vi "QMH_Tester_rev1.vi"() -> ()   [LabVIEW 2015]
doc: "Demonstrates the fundamentals of the Queued Message Handler design pattern in LabVIEW. A queued message handler, in its simplest form, is composed of two loops. The Event Handling Loop responds to user interface events by enqueuing \"messages\" on a message queue. These messages are dequeued in the Message Handling Loop. Note that the Message Handling Loop is also capable of sending messages to itself."
uses:
  Controls/Control_Stop.ctl
  Controls/Control_Unitherm Connect Disconnect Bool.ctl
  Controls/Control_M4X Connect Disconnect Bool.ctl
  Controls/Control_Fornax Connect Disconnect Bool.ctl
  Controls/Control_Unitherm Set Load Numeric.ctl
  Controls/Control_Unitherm Set Load Bool.ctl
  Controls/Control_Unitherm VISA Resource.ctl
  Controls/Control_Unitherm Clear Load Bool.ctl
  Controls/Control_PXI-7854R Connect Disconnect Bool.ctl
  Controls/Control_PXI-7854R 75kHz Bool.ctl
  Controls/Control_PXI-7854R uSec Off Numeric.ctl
  Controls/Control_PXI-7854R uSec On Numeric.ctl
  Controls/Control_PXI-7854R Resource.ctl
  Controls/Control_PXI-7854R Set Config Bool.ctl
  Controls/Control_PXI-7854R Set Config Enum.ctl
  Controls/Control_M4X Read Current Bool.ctl
  Controls/Control_Log Bool.ctl
  Controls/Control_Fornax Ligasure Activate Port Bool.ctl
  Controls/Control_Fornax Bipolar Activate Port Bool.ctl
  Controls/Control_Fornax Bipolar Decrease Power.ctl
  Controls/Control_Fornax Bipolar Increase Power.ctl
  Controls/Control_Fornax Bipolar Enum.ctl
  Controls/Control_Fornax Mono1 Cut Activate Port Bool.ctl
  Controls/Control_Fornax Mono1 Cut Enum.ctl
  Controls/Control_Fornax Mono1 Cut Increase Power.ctl
  Controls/Control_Fornax Mono1 Cut Decrease Power.ctl
  Controls/Control_Fornax Mono1 Coag Enum.ctl
  Controls/Control_Fornax Mono1 Coag Activate Port Bool.ctl
  Controls/Control_Fornax Mono1 Coag Increase Power.ctl
  Controls/Control_Fornax Mono1 Coag Decrease Power.ctl
  Controls/Control_Fornax Mono2 Cut Activate Port Bool.ctl
  Controls/Control_Fornax Mono2 Cut Increase Power.ctl
  Controls/Control_Fornax Mono2 Cut Decrease Power.ctl
  Controls/Control_Fornax Mono2 Cut Enum.ctl
  Controls/Control_Fornax Mono2 Coag Activate Port Bool.ctl
  Controls/Control_Fornax Mono2 Coag Enum.ctl
  Controls/Control_Fornax Mono2 Coag Increase Power.ctl
  Controls/Control_Fornax Mono2 Coag Decrease Power.ctl
  Controls/QMH Fundamentals - Message Cluster.ctl
  Controls/Control_Message Handling Cluster.ctl
  Controls/Control_M4X Connection.ctl
  Controls/Control_PXI-7854R FPGA Reference.ctl
  Controls/Control_Config Cluster.ctl
  Controls/Control_Config Unitherm Port.ctl
  Controls/Control_Config Simulate Values.ctl
  Controls/Control_Log Queue.ctl
  Controls/Control_Log Cluster.ctl
  Controls/Control_Log Time.ctl
  Controls/Control_Log Waveform Cluster.ctl
  Controls/Control_Log Analysis Cluster.ctl
  Controls/Control_Log Flag.ctl
  Controls/Config_Stop Notifier Enum.ctl
  Controls/Control_Log Loop Cluster.ctl
  Controls/Control_Log TDMS Filename.ctl
  Controls/Control_Log t0.ctl
  Controls/Control_Unitherm Connect Disconnect Cluster.ctl
  Controls/Control_PXI-7854R Connect Disconnect Cluster.ctl
  Controls/Control_PXI-7854R Set Config Cluster.ctl
  Controls/Control_Fornax Generator.ctl
  Controls/Control_Fornax Energy Channel ID.ctl
  Controls/Control_Fornax Instrument Type.ctl
  Controls/Control_Fornax Parameter Type.ctl
  Controls/Control_Fornax Parameter Value.ctl
  Controls/Control_Fornax Energy Mode.ctl
  <vilib>/Utility/error.llb/Error Cluster From Error Code.vi
  <vilib>/rvi/errors/niLvFpgaAdjustHostInterfaceError.vi
  <vilib>/rvi/interface/nirviReadWriteControl/nirviReadWriteControl.xnode
  <vilib>/ErrorRing/Error Ring.xnode
  NiFpgaLv.dll
  <vilib>/rvi/interface/Simulation/niFpgaSimulationCallBeginRW.vi
panel:
  in  "Mono2 Coag minus":T1
  in  "Mono2 Coag plus":T2
  in  "Mono2 Coag Enum":T3=enum."Spray"
  in  "Mono2 Coag Activate":T4
  in  "Mono2 Cut Enum":T5
  in  "Mono2 Cut minus":T6
  in  "Mono2 Cut plus":T7
  in  "Mono2 Cut Activate":T8
  in  "Mono1 Coag minus":T9
  in  "Mono1 Coag plus":T10
  in  "Mono1 Coag Activate":T11
  in  "Mono1 Coag Enum":T12=enum."Spray"
  in  "Mono1 Cut minus":T13
  in  "Mono1 Cut plus":T14
  in  "Mono1 Cut Enum":T15
  in  "Mono1 Cut Activate":T16
  in  "Bipolar Enum":T17
  in  "Bipolar plus":T18
  in  "Bipolar minus":T19
  in  "Bipolar Activate":T20
  in  "Ligasure Activate":T21
  out "Logging?":bool
  in  "Log?":T22
  out "Data":waveform(dbl)[](graph)
  out "Array":T23(array[cluster])
  in  "Read Current":T24
  in  "7854 Config Enum":T25=enum."Off"
  in  "7854 Set Config":T26
  in  "resource name":T27="PXI1Slot6" caption="RIO Device"
  in  "uSec On":T28=7
  in  "uSec Off":T29=6
  in  "75kHz":T30=TRUE
  in  "7854 Connect/Disconnect":T31
  out "PXI-7854R Connected?":bool
  in  "Clear Load":T32
  in  "Unitherm Refnum in":T33="COM4"
  in  "Set Load":T34
  in  "Load (Ohms)":T35
  out "M4X Connected?":bool
  in  "Fornax Connect/Disconnect":T36
  in  "M4X Connect/Disconnect":T37
  in  "Unitherm Connect/Disconnect":T38
  out "Unitherm Connected?":bool
  out "Fornax Connected?":bool
  out "Display Message":string="\"Stop\" button pressed"
  in  "Stop":T39
  # "Unitherm"
  # "PXI-7854R"
  # "M4X"
  # "Note: If you are creating a LabVIEW application based on the Queued Message Handler design pattern, create a Queued Message Handler project from the File > Create Project dialog."
  # "Fornax"
  # "Mono1"
  # "Mono2"
  # "Bipolar"
  # "Ligasure"
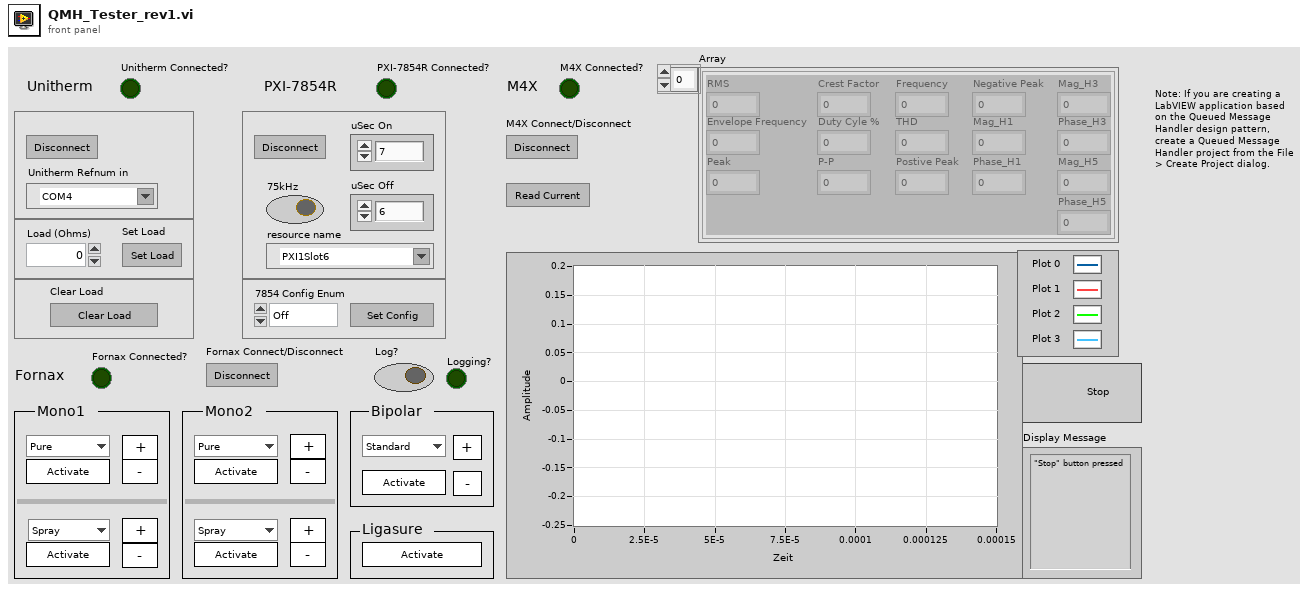
[diagram p1: front panel]
types:
  T1 = typedef "Control_Fornax Mono2 Coag Decrease Power.ctl" = bool
  T2 = typedef "Control_Fornax Mono2 Coag Increase Power.ctl" = bool
  T3 = typedef "Control_Fornax Mono2 Coag Enum.ctl" = enum16{"Fulgerate", "Spray"}
  T4 = typedef "Control_Fornax Mono2 Coag Activate Port Bool.ctl" = bool
  T5 = typedef "Control_Fornax Mono2 Cut Enum.ctl" = enum16{"Pure", "Blend"}
  T6 = typedef "Control_Fornax Mono2 Cut Decrease Power.ctl" = bool
  T7 = typedef "Control_Fornax Mono2 Cut Increase Power.ctl" = bool
  T8 = typedef "Control_Fornax Mono2 Cut Activate Port Bool.ctl" = bool
  T9 = typedef "Control_Fornax Mono1 Coag Decrease Power.ctl" = bool
  T10 = typedef "Control_Fornax Mono1 Coag Increase Power.ctl" = bool
  T11 = typedef "Control_Fornax Mono1 Coag Activate Port Bool.ctl" = bool
  T12 = typedef "Control_Fornax Mono1 Coag Enum.ctl" = enum16{"Fulgerate", "Spray"}
  T13 = typedef "Control_Fornax Mono1 Cut Decrease Power.ctl" = bool
  T14 = typedef "Control_Fornax Mono1 Cut Increase Power.ctl" = bool
  T15 = typedef "Control_Fornax Mono1 Cut Enum.ctl" = enum16{"Pure", "Blend"}
  T16 = typedef "Control_Fornax Mono1 Cut Activate Port Bool.ctl" = bool
  T17 = typedef "Control_Fornax Bipolar Enum.ctl" = enum16{"Standard", "Macro", "Precision"}
  T18 = typedef "Control_Fornax Bipolar Increase Power.ctl" = bool
  T19 = typedef "Control_Fornax Bipolar Decrease Power.ctl" = bool
  T20 = typedef "Control_Fornax Bipolar Activate Port Bool.ctl" = bool
  T21 = typedef "Control_Fornax Ligasure Activate Port Bool.ctl" = bool
  T22 = typedef "Control_Log Bool.ctl" = bool
  T23 = cluster{"RMS":dbl, "Envelope Frequency":dbl, "Peak":dbl, "Crest Factor":dbl, "Duty Cyle %":dbl, "P-P":dbl, "Frequency":dbl, "THD":dbl, "Postive Peak":dbl, "Negative Peak":dbl, "Mag_H1":dbl, "Phase_H1":dbl, "Mag_H3":dbl, "Phase_H3":dbl, "Mag_H5":dbl, "Phase_H5":dbl}[]
  T24 = typedef "Control_M4X Read Current Bool.ctl" = bool
  T25 = typedef "Control_PXI-7854R Set Config Enum.ctl" = enum16{"Mono 1", "Mono 2", "BiPolar", "LigaSure", "Off"}
  T26 = typedef "Control_PXI-7854R Set Config Bool.ctl" = bool
  T27 = typedef "Control_PXI-7854R Resource.ctl" = tag
  T28 = typedef "Control_PXI-7854R uSec On Numeric.ctl" = u16
  T29 = typedef "Control_PXI-7854R uSec Off Numeric.ctl" = u16
  T30 = typedef "Control_PXI-7854R 75kHz Bool.ctl" = bool
  T31 = typedef "Control_PXI-7854R Connect Disconnect Bool.ctl" = bool
  T32 = typedef "Control_Unitherm Clear Load Bool.ctl" = bool
  T33 = typedef "Control_Unitherm VISA Resource.ctl" = refnum<visa-resource-name>
  T34 = typedef "Control_Unitherm Set Load Bool.ctl" = bool
  T35 = typedef "Control_Unitherm Set Load Numeric.ctl" = i32
  T36 = typedef "Control_Fornax Connect Disconnect Bool.ctl" = bool
  T37 = typedef "Control_M4X Connect Disconnect Bool.ctl" = bool
  T38 = typedef "Control_Unitherm Connect Disconnect Bool.ctl" = bool
  T39 = typedef "Control_Stop.ctl" = bool
  T40 = typedef "Control_Log Loop Cluster.ctl" = cluster{"tdms file out":T41, "t0":T42}
  T41 = typedef "Control_Log TDMS Filename.ctl" = refnum<k34>
  T42 = typedef "Control_Log t0.ctl" = string
  T43 = typedef "Config_Stop Notifier Enum.ctl" = enum16{"Initialize", "Read Notifier", "Notify", "Close"}
  T44 = typedef "Control_Log Cluster.ctl" = cluster{"Log Time":T45, "Log Waveform Cluster":T46, "Log Analysis Cluster":T47}
  T45 = typedef "Control_Log Time.ctl" = timestamp
  T46 = typedef "Control_Log Waveform Cluster.ctl" = waveform(dbl)
  T47 = typedef "Control_Log Analysis Cluster.ctl" = cluster{"RMS":dbl, "Envelope Frequency":dbl, "Peak":dbl, "Crest Factor":dbl, "Duty Cyle %":dbl, "P-P":dbl, "Frequency":dbl, "THD":dbl, "Postive Peak":dbl, "Negative Peak":dbl, "Mag_H1":dbl, "Phase_H1":dbl, "Mag_H3":dbl, "Phase_H3":dbl, "Mag_H5":dbl, "Phase_H5":dbl}
  T48 = typedef "Control_Message Handling Cluster.ctl" = cluster{"Fornax Connected?":refnum<vi>, "Unitherm Connected?":refnum<vi>, "M4X Connected?":refnum<vi>, "Unitherm Connect/Disconnect":refnum<vi>, "Fornax Connection":refnum<k5>, "UNITHERM Connection":refnum<visa-resource-name>, "M4X Connection":T49, "PXI-7854R FPGA Reference":T50, "PXI-7854R Connected?":refnum<vi>, "Fornax Connect/Disconnect":refnum<vi>, "7854 Connect/Disconnect":refnum<vi>, "M4X Connect/Disconnect":refnum<vi>, "Config Cluster":T51, "Log Queue":T54, "Log Analysis Cluster":T47, "Log Waveform Cluster":T46, "Log Time":T45, "Log Flag":T55}
  T49 = typedef "Control_M4X Connection.ctl" = u32
  T50 = typedef "Control_PXI-7854R FPGA Reference.ctl" = refnum<k20>
  T51 = typedef "Control_Config Cluster.ctl" = cluster{"Unitherm Port":T52, "Simulate Values":T53}
  T52 = typedef "Control_Config Unitherm Port.ctl" = string
  T53 = typedef "Control_Config Simulate Values.ctl" = bool
  T54 = typedef "Control_Log Queue.ctl" = refnum<queue>
  T55 = typedef "Control_Log Flag.ctl" = bool
  T56 = typedef "QMH Fundamentals - Message Cluster.ctl" = cluster{"Message":string, "Message Data":variant}
  T57 = typedef "Control_Unitherm Connect Disconnect Cluster.ctl" = cluster{"Unitherm Connect/Disconnect":T38, "Unitherm Refnum in":T33}
  T58 = typedef "Control_PXI-7854R Connect Disconnect Cluster.ctl" = cluster{"PXI-7854R Resource":T27, "75kHz":T30, "uSec Off":T29, "uSec On":T28, "7854 Connect/Disconnect":T31}
  T59 = typedef "Control_PXI-7854R Set Config Cluster.ctl" = cluster{"7854 Config Enum":T25, "7854 Set Config":T26}
  T60 = typedef "Control_Fornax Energy Mode.ctl" = enum16{"SPRAY_MODE", "CUT_MODE", "BLEND_MODE", "FULGERATE_MODE", "BIPOLAR_MODE", "VESSEL_SEALING_MODE", "VALLEYLAB_MODE", "BIPOLAR_RESECTION_CUT_MODE", "BIPOLAR_RESECTION_COAG_MODE", "AUTOBIPOLAR_MODE", "VIPER_HLA", "SOFT_COAG_MODE", "ECUT_MODE", "SHARED_SPRAY_MODE", "SHARED_FULGERATE_MODE", "CARDIO_MONO_MODE", "CARDIO_BIPOLAR_MODE", "BIPOLAR_LOW_MODE", "BIPOLAR_MACRO_MODE", "BIPOLAR_STANDARD_MODE", "BIPOLAR_MEDIUM_MODE", "VL_ENDOSCOPY_MODE", "NUM_ENERGY_MODES"}
  T61 = typedef "Control_Fornax Parameter Value.ctl" = i32
  T62 = typedef "Control_Fornax Parameter Type.ctl" = enum16{"POWER_PARAMETER", "CUT_MODALITY_POWER_PARAMETER", "COAG_MODALITY_POWER_PARAMETER", "VL_MODALITY_POWER_PARAMETER", "BY_MODE_POWER_PARAMETER", "VL_ENDO_CUT_MODALITY_POWER_PARAMETER", "VL_ENDO_COAG_MODALITY_POWER_PARAMETER", "VL_ENDO_COAG_ON_CUT_MODALITY_POWER_PARAMETER", "MODE_PARAMETER   (for changing Bipolar mode)", "CUT_MODALITY_MODE_PARAMETER  (for changing monopolar cut mode)", "COAG_MODALITY_MODE_PARAMETER (for changing monopolar coag mode)", "VL_ENDO_COAG_MODALITY_MODE_PARAMETER", "VL_ENDO_CUT_INTERVAL_PARAMETER", "VL_ENDO_CUT_DURATION_PARAMETER", "POWER_BAR_PARAMETER", "MAX_ACTIVATION_MSEC_TIME_PARAMETER", "AUTOBIPOLAR_DELAY_MSEC_TIME", "VL_ENDO_COAG_QUICK_ACCESS_PARAMETER"}
  T63 = typedef "Control_Fornax Instrument Type.ctl" = enum16{"INSTRUMENT_TYPE_UNKNOWN", "INSTRUMENT_TYPE_MONOPOLAR", "INSTRUMENT_TYPE_BIPOLAR", "INSTRUMENT_TYPE_TRIVERSE", "INSTRUMENT_TYPE_LIGASURE", "INSTRUMENT_TYPE_ADVANCE_II", "INSTRUMENT_TYPE_BIPOLAR_RESECTION", "INSTRUMENT_TYPE_HOOK", "INSTRUMENT_TYPE_BIZACT", "INSTRUMENT_TYPE_CARDIOBLATE_BIP", "INSTRUMENT_TYPE_CARDIOBLATE_BIP_GEMINI_S", "INSTRUMENT_TYPE_CARDIOBLATE_MONO", "INSTRUMENT_TYPE_ULTRASONIC", "INSTRUMENT_TYPE_MONOPOLAR_GI ", "INSTRUMENT_TYPE_GOLDILOCKS "}
  T64 = typedef "Control_Fornax Energy Channel ID.ctl" = enum16{"EC_MONO_1  ", "EC_BIPOLAR  ", "EC_MONO_2  ", "EC_ADVANCED  ", "EC_ADVANCED_ECUT  ", "EC_ADVANCED_DCUT  ", "EC_SHARED_COAG  ", "EC_INTERNAL_BIP_CAL  "}
  T65 = typedef "Control_Fornax Generator.ctl" = string
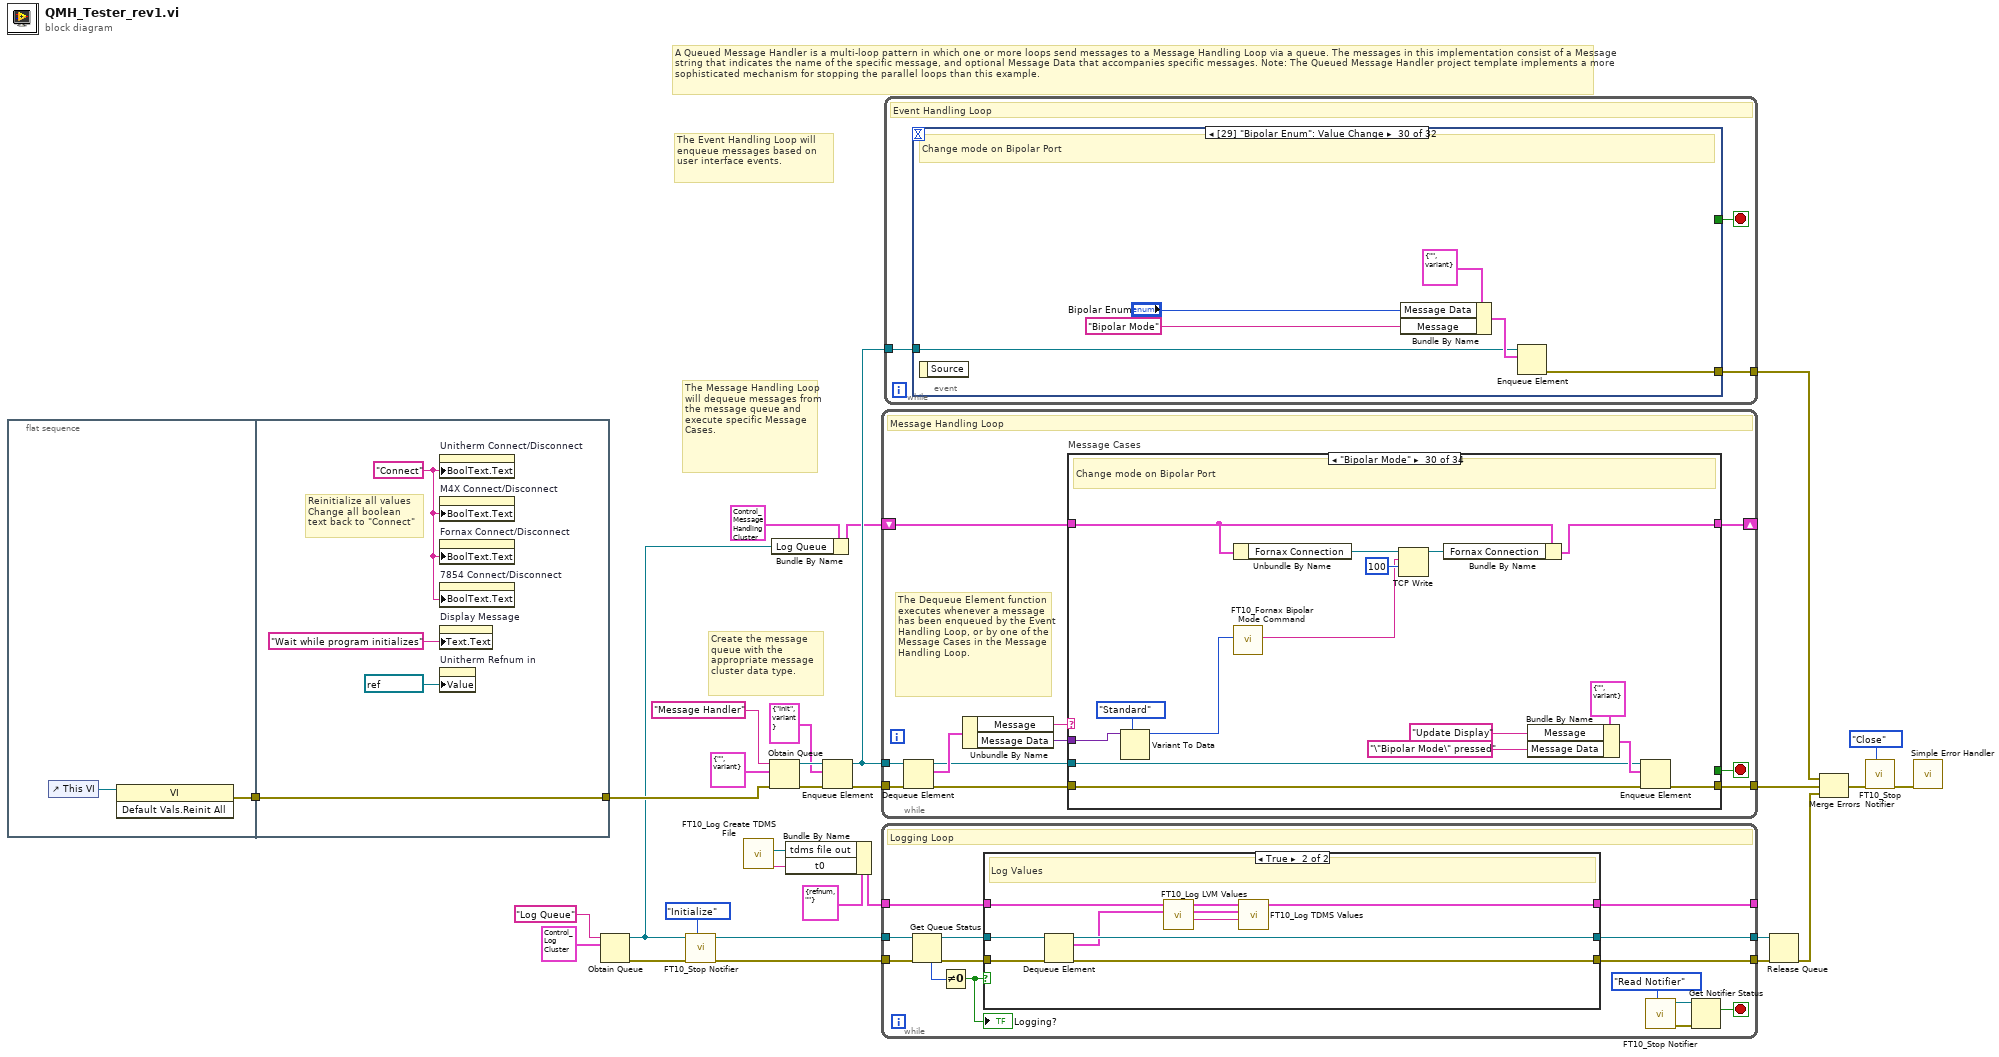
[diagram p0: block diagram]
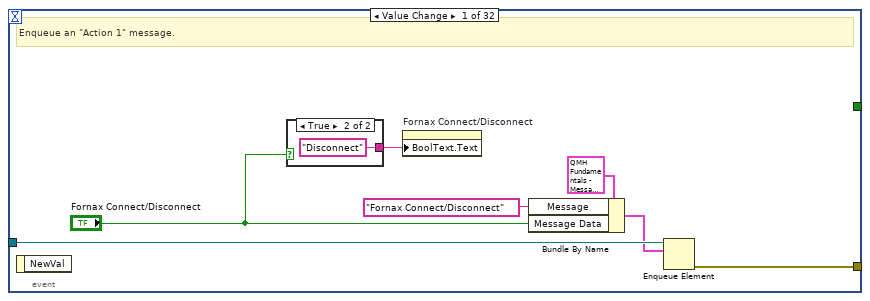
[diagram p3: hidden frame]
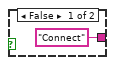
[diagram p4: hidden frame]
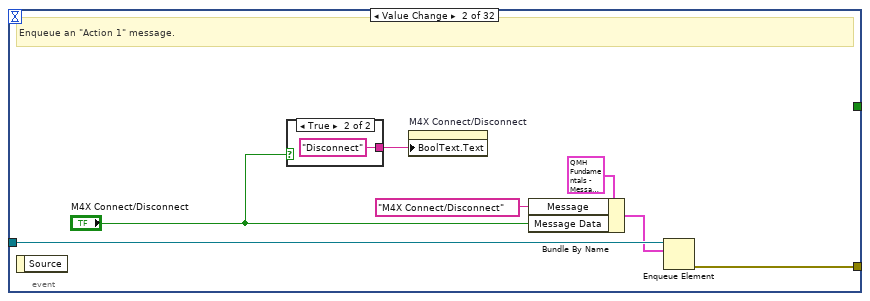
[diagram p5: hidden frame]
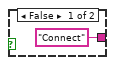
[diagram p6: hidden frame]
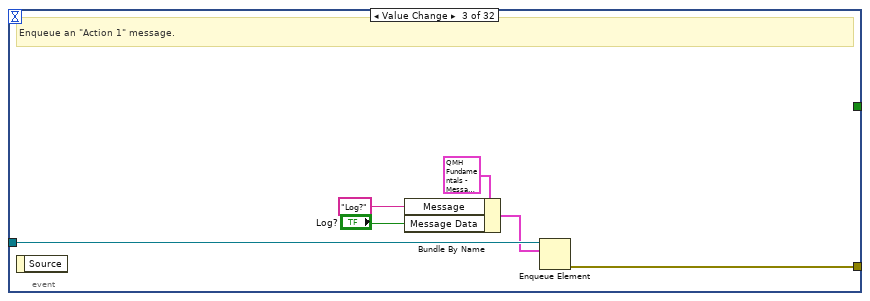
[diagram p7: hidden frame]
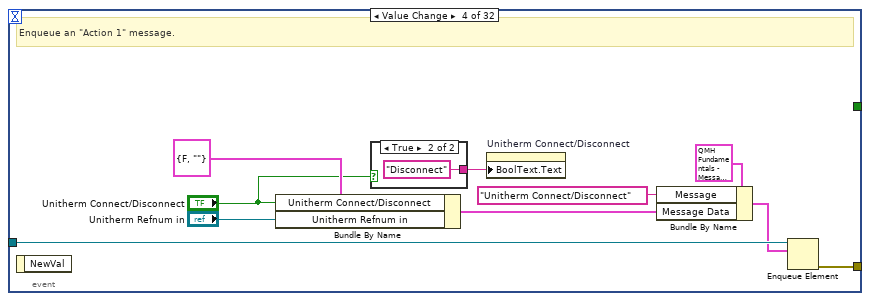
[diagram p8: hidden frame]
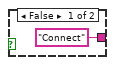
[diagram p9: hidden frame]
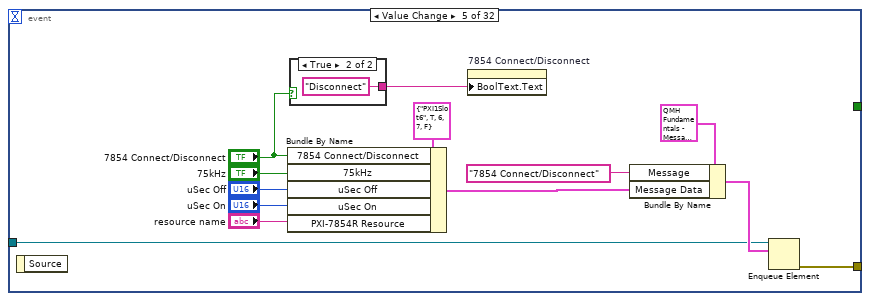
[diagram p10: hidden frame]
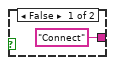
[diagram p11: hidden frame]
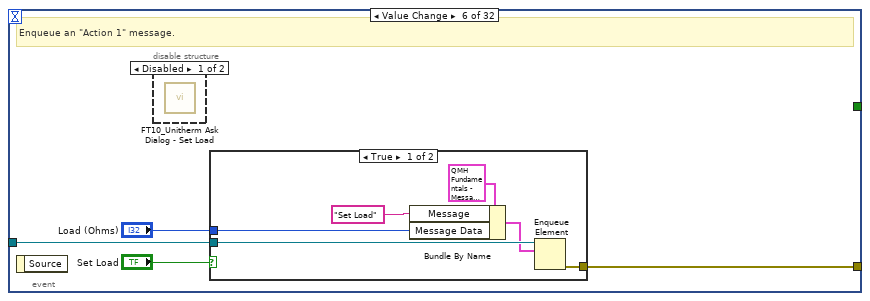
[diagram p12: hidden frame]
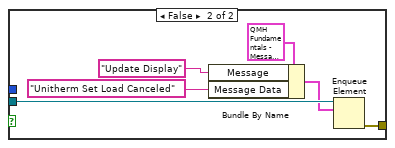
[diagram p14: hidden frame]
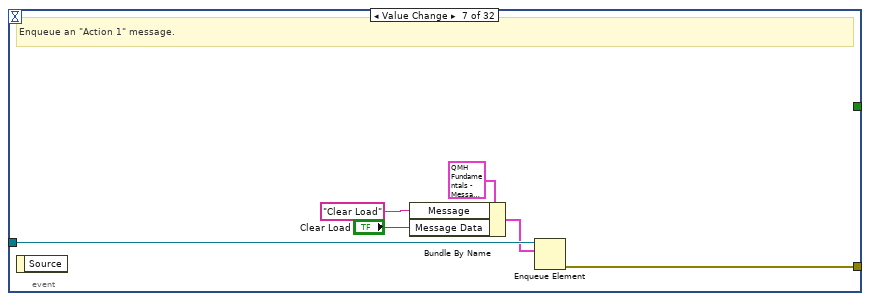
[diagram p15: hidden frame]
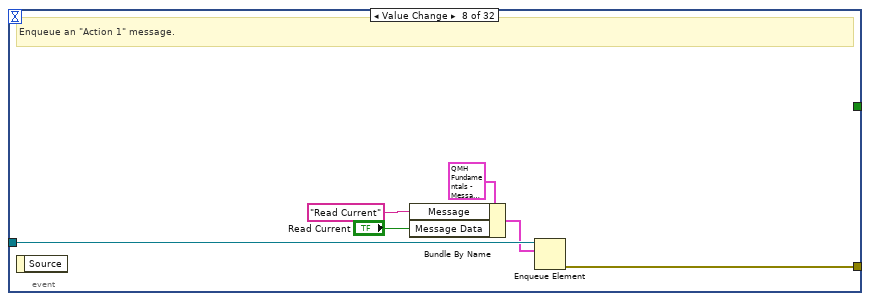
[diagram p16: hidden frame]
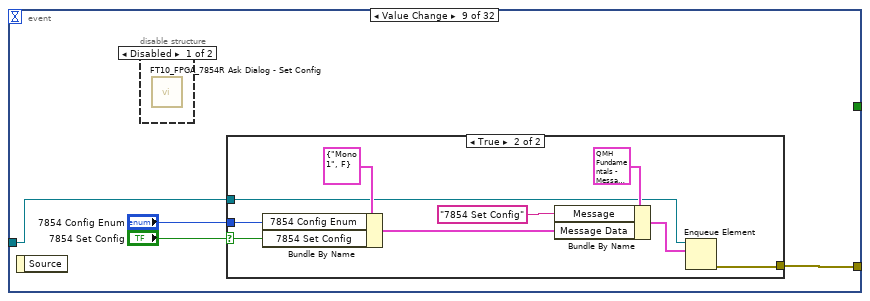
[diagram p17: hidden frame]
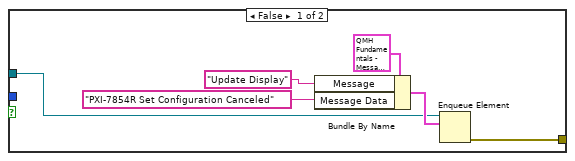
[diagram p19: hidden frame]
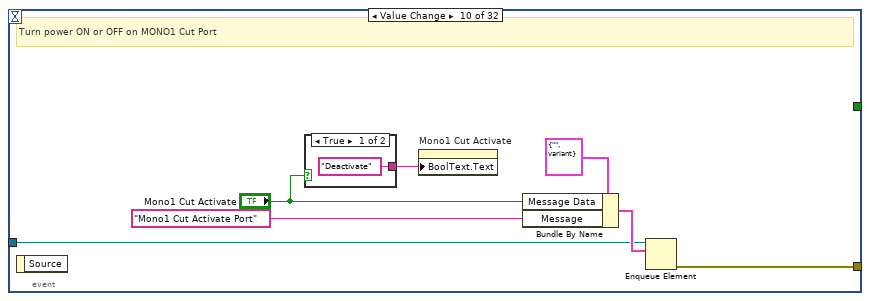
[diagram p20: hidden frame]
diagram:
  # "Create the message queue with the appropriate message cluster data type."
  # "A Queued Message Handler is a multi-loop pattern in which one or more loops send messages to a Message Handling Loop via a queue. The messages in this implementation consist of a Message string that indicates the name of the specific message, and optional Message Data that accompanies specific messages. Note: The Queued Message Handler project template implements a more sophisticated mechanism for stopping the parallel loops than this example."
  # "The Message Handling Loop will dequeue messages from the message queue and execute specific Message Cases."
  # "The Event Handling Loop will enqueue messages based on user interface events."
  n1 = flat-sequence {
    tunnel: [w30] -> w18
    tunnel: [w35] -> w21
    tunnel: w18 -> [w35]
    frame #0 {
      n2 = control-ref of="This VI"() -> (w31:refnum<vi>)
      n3 = invoke class="VI" method="Default Vals.Reinit All"(reference=w31) -> (error out=w30:errorcluster)  [unwired: 2 in, 2 out]
    }
    frame #1 {
      w33 = "Connect" ("Boolean Text.Text")
      # "Reinitialize all values\nChange all boolean\ntext back to \"Connect\""
      n4 = property on="Unitherm Connect/Disconnect" class="Bool (strict)"("BoolText.Text"=w33) -> ()  [unwired: 2 in, 2 out]
      n5 = property on="M4X Connect/Disconnect" class="Bool (strict)"("BoolText.Text"=w33) -> ()  [unwired: 2 in, 2 out]
      n6 = property on="Fornax Connect/Disconnect" class="Bool (strict)"("BoolText.Text"=w33) -> ()  [unwired: 2 in, 2 out]
      n7 = property on="7854 Connect/Disconnect" class="Bool (strict)"("BoolText.Text"=w33) -> ()  [unwired: 2 in, 2 out]
      n8 = property on="Display Message" class="Str"("Text.Text"="Wait while program initializes" ("Display Message")) -> ()  [unwired: 2 in, 2 out]
      n9 = property on="Unitherm Refnum in" class="VISAName (strict)"("Value"=refnum<visa-resource-name> "COM4" ("Unitherm Refnum in")) -> ()  [unwired: 2 in, 2 out]
    }
  }
  n10 = Obtain Queue(name (unnamed)="Log Queue", element data type=T44 {"Log Time"=timestamp(0 s since 1904-01-01), "Log Waveform Cluster"={"t0"=timestamp(0 s since 1904-01-01), "dt"=1.0, "Y"=[]}, "Log Analysis Cluster"={"RMS"=0.0, "Envelope Frequency"=0.0, "Peak"=0.0, "Crest Factor"=0.0, "Duty Cyle %"=0.0, "P-P"=0.0, "Frequency"=0.0, "THD"=0.0, "Postive Peak"=0.0, "Negative Peak"=0.0, "Mag_H1"=0.0, "Phase_H1"=0.0, "Mag_H3"=0.0, "Phase_H3"=0.0, "Mag_H5"=0.0, "Phase_H5"=0.0}}) -> (queue out=w11:refnum<queue>, error out=w9:errorcluster)  [unwired: 3 in, 1 out]
  n11 = call "FT10_Stop Notifier.vi"("Selector"=Config_Stop_Notifier_Enum."Initialize", "error in (no error)"=w9) -> ("error out"=w8:errorcluster)  [unwired: 8 in, 1 out]
  n12 = call "FT10_Log Create TDMS File.vi"() -> ("t0"=w2:T42, "tdms file out"=w1:T41)  [unwired: 10 in]
  n13 = Obtain Queue(name (unnamed)="Message Handler", element data type=T56 {"Message"="", "Message Data"=variant} ("Message Cluster"), error in (no error)=w21) -> (queue out=w25:refnum<queue>, error out=w26:errorcluster)  [unwired: 2 in, 1 out]
  n14 = Bundle By Name(cluster=T48 {"Fornax Connected?"=refnum, "Unitherm Connected?"=refnum, "M4X Connected?"=refnum, "Unitherm Connect/Disconnect"=refnum, "Fornax Connection"=refnum, "UNITHERM Connection"="", "M4X Connection"=0, "PXI-7854R FPGA Reference"=refnum, "PXI-7854R Connected?"=refnum, "Fornax Connect/Disconnect"=refnum, "7854 Connect/Disconnect"=refnum, "M4X Connect/Disconnect"=refnum, "Config Cluster"={"Unitherm Port"="COM4", "Simulate Values"=TRUE}, "Log Queue"=refnum, "Log Analysis Cluster"={"RMS"=0.0, "Envelope Frequency"=0.0, "Peak"=0.0, "Crest Factor"=0.0, "Duty Cyle %"=0.0, "P-P"=0.0, "Frequency"=0.0, "THD"=0.0, "Postive Peak"=0.0, "Negative Peak"=0.0, "Mag_H1"=0.0, "Phase_H1"=0.0, "Mag_H3"=0.0, "Phase_H3"=0.0, "Mag_H5"=0.0, "Phase_H5"=0.0}, "Log Waveform Cluster"={"t0"=timestamp(0 s since 1904-01-01), "dt"=1.0, "Y"=[]}, "Log Time"=timestamp(0 s since 1904-01-01), "Log Flag"=FALSE}, "Log Queue"=w11) -> (w12:T48)
  n15 = Bundle By Name(cluster=T40 {"tdms file out"=refnum, "t0"=""}, "tdms file out"=w1, "t0"=w2) -> (w3:T40)
  n16 = Enqueue Element(queue=w25, element=T56 {"Message"="Init", "Message Data"=variant}, error in (no error)=w26) -> (queue out=w19:refnum<queue>, error out=w24:errorcluster)  [unwired: 1 in, 1 out]
  n17 = while {
    tunnel: w19 -> [w45]
    tunnel: w24 -> [w46]
    tunnel: [w38] -> w29
    shift-right: [w39] -> _
    shift-left: w12 -> [w36]
    stop <- w37 stop-if-true
    # "The Dequeue Element function executes whenever a message has been enqueued by the Event Handling Loop, or by one of the Message Cases in the Message Handling Loop."
    # "Message Handling Loop"
    n18 = Dequeue Element(queue=w45, error in (no error)=w46) -> (queue out=w43:refnum<queue>, element=w44:T56, error out=w42:errorcluster)  [unwired: 1 in, 1 out]
    n19 = Unbundle By Name(w44) -> ("Message"=w41:string, "Message Data"=w40:variant)
    n20 = case "Message Cases" shown="\"Bipolar Mode\"" w41 {
      selector: w41 -> [_ _ _ _ _ _ _ _ _ _ _ _ _ _ _ _ _ _ _ _ _ _ _ _ _ _ _ _ _ _ _ _ _ w610]
      tunnel: w43 -> [w68 w85 w104 w133 w152 w177 w190 w203 w204 w232 w246 w260 w274 w288 w302 w321 w340 w359 w378 w397 w416 w435 w454 w473 w492 w508 w524 w540 w556 w572 _ _ w604 _]
      tunnel: w42 -> [w47 w84 w95 w124 w143 w163 w179 w195 w207 w231 w245 w259 w273 w287 w301 w320 w339 w358 w377 w396 w415 w434 w453 w472 w491 w507 w523 w539 w555 w571 w582 w588 w596 w609]
      tunnel: [w69 w86 w105 w134 w153 w169 w183 w197 w208 w230 w244 w258 w272 w286 w300 w319 w338 w357 w376 w395 w414 w433 w452 w471 w490 w506 w522 w538 w554 w570 w582 w585 w589 w609] -> w38
      tunnel: w40 -> [_ w79 w102 w123 w144 w167 _ _ w216 w227 w242 w256 w268 w282 w296 _ _ _ _ _ _ _ _ _ _ w499 w515 w530 w547 w563 w581 w587 _ _]
      tunnel: w36 -> [w67 w90 w97 w128 w146 w170 w184 w198 w219 w229 w243 w257 w271 w285 w299 w318 w337 w356 w375 w394 w413 w432 w451 w470 w489 w505 w521 w537 w553 w569 w580 w583 w599 w607]
      tunnel: [w62 w83 w96 w127 w145 w171 w185 w191 w218 w223 w241 w255 w270 w284 w298 w317 w336 w355 w374 w393 w412 w431 w450 w469 w488 w504 w520 w536 w552 w568 w579 w583 w598 w607] -> w39
      tunnel: [_ _ _ _ _ _ _ _ _ _ _ _ _ _ _ _ _ _ _ _ _ _ _ _ _ _ _ _ _ _ _ _ TRUE _] -> w37
      frame "Init" {
        # "Initialize - Create reference for connection indicators. Connect to Fornax, M4X, and Unitherm."
        n21 = call "FT10_Config Parse File.vi"("error in (no error)"=w47, "File Path Control"=path "Config.ini") -> ("error out"=w49:errorcluster, "Config cluster"=w48:T51)  [unwired: 8 in]
        n22 = control-ref of="Fornax Connected?"() -> (w66:refnum<vi>)
        n23 = control-ref of="Unitherm Connected?"() -> (w65:refnum<vi>)
        n24 = control-ref of="M4X Connected?"() -> (w64:refnum<vi>)
        n25 = control-ref of="PXI-7854R Connected?"() -> (w56:refnum<vi>)
        n26 = control-ref of="Unitherm Connect/Disconnect"() -> (w54:refnum<vi>)
        n27 = control-ref of="Fornax Connect/Disconnect"() -> (w53:refnum<vi>)
        n28 = control-ref of="7854 Connect/Disconnect"() -> (w52:refnum<vi>)
        n29 = control-ref of="M4X Connect/Disconnect"() -> (w51:refnum<vi>)
        n30 = Bundle By Name(cluster=w67, "Fornax Connected?"=w66, "Unitherm Connected?"=w65, "M4X Connected?"=w64, "PXI-7854R Connected?"=w56, "UNITHERM Connection"=refnum<visa-resource-name> "COM4", "Unitherm Connect/Disconnect"=w54, "Fornax Connect/Disconnect"=w53, "7854 Connect/Disconnect"=w52, "M4X Connect/Disconnect"=w51, "Config Cluster"=w48) -> (w63:T48)
        n31 = Bundle By Name(cluster=T56 {"Message"="", "Message Data"=variant} ("Message Cluster"), "Message"="Update Display", "Message Data"="Initialize Complete" ("L10n_Action 1 Pressed")) -> (w72:T56)
        n32 = call "FT10_Connect Hardware.vi"("Message Handling Cluster in"=w63, "error in (no error)"=w49) -> ("Message Handling Cluster out"=w62:T48, "Fornax Connected?"=→"Fornax Connected?":bool, "Unitherm Connected?"=→"Unitherm Connected?":bool, "M4X Connected?"=→"M4X Connected?":bool, "PXI-7854R Connected?"=→"PXI-7854R Connected?":bool, "error out"=w61:errorcluster)  [unwired: 8 in]
        n33 = Enqueue Element(queue=w68, element=w72, error in (no error)=w47) -> (error out=w70:errorcluster)  [unwired: 1 in, 2 out]
        n34 = Merge Errors(w61, w70) -> (w69:errorcluster)
      }
      frame "Fornax Connect/Disconnect" {
        # "Connect or disconnect from Fornax."
        n35 = Variant To Data(type=TRUE, Variant=w79) -> (data=w76:bool)  [unwired: 1 in, 1 out]
        n36 = case shown="True" w76 {
          tunnel: ["Fornax Disconnect" ("L10n_Action 1 Pressed") "Fornax Connect" ("L10n_Action 1 Pressed")] -> w75
          frame False {
          }
          frame True {
          }
        }
        n37 = call "FT10_Connect Fornax Handler.vi"("error in (no error)"=w84, "Message Data"=w79, "Message Handling Cluster in"=w90) -> ("error out"=w81:errorcluster, "Fornax Connected?"=w80:bool, "Message Handling Cluster out"=w83:T48)  [unwired: 6 in]
        n38 = Bundle By Name(cluster=T56 {"Message"="", "Message Data"=variant} ("Message Cluster"), "Message Data"=w75, "Message"="Update Display") -> (w88:T56)
        n39 = Enqueue Element(queue=w85, element=w88, error in (no error)=w84) -> (error out=w87:errorcluster)  [unwired: 1 in, 2 out]
        n40 = Unbundle By Name(w83) -> ("Fornax Connected?"=w82:refnum<vi>)
        n41 = property class="Bool (strict)"(reference=w82, "Value"=w80) -> ()  [unwired: 1 in, 2 out]
        n42 = Merge Errors(w81, w87) -> (w86:errorcluster)
      }
      frame "M4X Connect/Disconnect" {
        # "Connect or disconnect from M4X."
        n43 = Variant To Data(type=TRUE, Variant=w102) -> (data=w99:bool)  [unwired: 1 in, 1 out]
        n44 = case shown="True" w99 {
          tunnel: ["M4X Disconnect" ("L10n_Action 1 Pressed") "M4X Connect" ("L10n_Action 1 Pressed")] -> w98
          tunnel: w97 -> [w111 w117]
          tunnel: [w111 w116] -> w96
          tunnel: w95 -> [w110 w115]
          tunnel: [w110 w114] -> w94
          tunnel: [FALSE ("M4X Connected?") w113] -> w93
          frame False {
          }
          frame True {
            n45 = call "FT10_Connect M4X.vi"("error in (no error)"=w115, "reset device"=TRUE, "Board #"=u32 0, "Message Handling Cluster in"=w117) -> ("error out"=w114:errorcluster, "M4X Connected?"=w113:bool, "Message Handling Cluster out"=w116:T48)  [unwired: 4 in, 1 out]
          }
        }
        n46 = Bundle By Name(cluster=T56 {"Message"="", "Message Data"=variant} ("Message Cluster"), "Message Data"=w98, "Message"="Update Display") -> (w107:T56)
        n47 = Enqueue Element(queue=w104, element=w107, error in (no error)=w95) -> (error out=w106:errorcluster)  [unwired: 1 in, 2 out]
        n48 = Unbundle By Name(w96) -> ("M4X Connected?"=w103:refnum<vi>)
        n49 = property class="Bool (strict)"(reference=w103, "Value"=w93) -> ()  [unwired: 1 in, 2 out]
        n50 = Merge Errors(w94, w106) -> (w105:errorcluster)
      }
      frame "Unitherm Connect/Disconnect" {
        # "Connect or disconnect from Unitherm."
        n51 = Variant To Data(type=T57 {"Unitherm Connect/Disconnect"=FALSE, "Unitherm Refnum in"=""}, Variant=w123) -> (data=w130:T57)  [unwired: 1 in, 1 out]
        n52 = Unbundle By Name(w130) -> ("Unitherm Connect/Disconnect"=w121:T38)
        n53 = call "FT10_Connect Unitherm Handler.vi"("error in (no error)"=w124, "Message Data"=w123, "Message Handling Cluster in"=w128) -> ("error out"=w125:errorcluster, "Unitherm Connected?"=w126:bool, "Message Handling Cluster out"=w127:T48)  [unwired: 6 in]
        n54 = case shown="False" w121 {
          tunnel: ["Unitherm Disconnect" ("L10n_Action 1 Pressed") "Unitherm Connect" ("L10n_Action 1 Pressed")] -> w129
          frame False {
          }
          frame True {
          }
        }
        n55 = Unbundle By Name(w127) -> ("Unitherm Connected?"=w132:refnum<vi>)
        n56 = Bundle By Name(cluster=T56 {"Message"="", "Message Data"=variant} ("Message Cluster"), "Message Data"=w129, "Message"="Update Display") -> (w136:T56)
        n57 = Enqueue Element(queue=w133, element=w136, error in (no error)=w124) -> (error out=w135:errorcluster)  [unwired: 1 in, 2 out]
        n58 = property class="Bool (strict)"(reference=w132, "Value"=w126) -> ()  [unwired: 1 in, 2 out]
        n59 = Merge Errors(w125, w135) -> (w134:errorcluster)
      }
      frame "7854 Connect/Disconnect" {
        # "Connect or disconnect from Unitherm."
        n60 = Variant To Data(type=T58 {"PXI-7854R Resource"="PXI1Slot6", "75kHz"=TRUE, "uSec Off"=6, "uSec On"=7, "7854 Connect/Disconnect"=FALSE}, Variant=w144) -> (data=w149:T58)  [unwired: 1 in, 1 out]
        n61 = Unbundle By Name(w149) -> ("7854 Connect/Disconnect"=w147:T31)
        n62 = case shown="False" w147 {
          tunnel: ["PXI-7854R Disconnected" ("L10n_Action 1 Pressed") "PXI-7854R Connected" ("L10n_Action 1 Pressed")] -> w148
          frame False {
          }
          frame True {
          }
        }
        n63 = call "FT10_Connect FPGA_7854R Handler.vi"("error in"=w143, "Message Data"=w144, "Message Handling Cluster in"=w146) -> ("error out"=w142:errorcluster, "PXI-7854R Connected?"=w141:bool, "Message Handling Cluster out"=w145:T48)  [unwired: 6 in]
        n64 = Unbundle By Name(w145) -> ("PXI-7854R Connected?"=w151:refnum<vi>)
        n65 = Bundle By Name(cluster=T56 {"Message"="", "Message Data"=variant} ("Message Cluster"), "Message Data"=w148, "Message"="Update Display") -> (w155:T56)
        n66 = Enqueue Element(queue=w152, element=w155, error in (no error)=w143) -> (error out=w154:errorcluster)  [unwired: 1 in, 2 out]
        n67 = property class="Bool (strict)"(reference=w151, "Value"=w141) -> ()  [unwired: 1 in, 2 out]
        n68 = Merge Errors(w142, w154) -> (w153:errorcluster)
      }
      frame "Set Load" {
        # "Adjust the Impedance of the Unitherm."
        n69 = Variant To Data(type=0 ("Load (Ohms)"), Variant=w167) -> (data=w162:i32)  [unwired: 1 in, 1 out]
        n70 = Number To Decimal String(number=w162) -> (decimal integer string=w160:string)  [unwired: 1 in]
        n71 = Unbundle By Name(w170) -> ("UNITHERM Connection"=w166:refnum<visa-resource-name>)
        n72 = Concatenate Strings("Unitherm Load set to " ("L10n_Action 1 Pressed"), w160, " Ohms" ("string")) -> (w161:string)
        n73 = call "FT10_Unitherm Set Load.vi"("error in (no error)"=w163, "Load Impedance"=w162, "VISA Refnum in"=w166) -> ("error out"=w164:errorcluster, "VISA Refnum out"=w165:refnum<visa-resource-name>)  [unwired: 7 in]
        n74 = Bundle By Name(cluster=T56 {"Message"="", "Message Data"=variant} ("Message Cluster"), "Message"="Update Display", "Message Data"=w161) -> (w173:T56)
        n75 = Bundle By Name(cluster=w170, "UNITHERM Connection"=w165) -> (w171:T48)
        n76 = Enqueue Element(queue=w177, element=w173, error in (no error)=w163) -> (error out=w176:errorcluster)  [unwired: 1 in, 2 out]
        n77 = Merge Errors(w164, w176) -> (w169:errorcluster)
      }
      frame "Clear Load" {
        # "Adjust the Impedance of the Unitherm."
        n78 = Unbundle By Name(w184) -> ("UNITHERM Connection"=w181:refnum<visa-resource-name>)
        n79 = call "FT10_Unitherm Clear Load.vi"("error in (no error)"=w179, "VISA Refnum in"=w181) -> ("error out"=w178:errorcluster, "VISA Refnum out"=w180:refnum<visa-resource-name>)  [unwired: 8 in]
        n80 = Bundle By Name(cluster=T56 {"Message"="", "Message Data"=variant} ("Message Cluster"), "Message"="Update Display", "Message Data"="Unitherm Load Cleared" ("L10n_Action 1 Pressed")) -> (w186:T56)
        n81 = Bundle By Name(cluster=w184, "UNITHERM Connection"=w180) -> (w185:T48)
        n82 = Enqueue Element(queue=w190, element=w186, error in (no error)=w179) -> (error out=w189:errorcluster)  [unwired: 1 in, 2 out]
        n83 = Merge Errors(w178, w189) -> (w183:errorcluster)
      }
      frame "Read Current" {
        # "Read data from M4X and send to logging loop if logging is enabled."
        n84 = call "FT10_M4X Read.vi"("Message Handling Cluster in"=w198) -> ("Waveform Array"=→"Data":waveform(dbl)[], "Analysis Cluster Array"=→"Array":T23, "Message Handling Cluster out"=w192:T48)  [unwired: 8 in]
        n85 = Bundle By Name(cluster=T56 {"Message"="", "Message Data"=variant} ("Message Cluster"), "Message"="Update Display", "Message Data"="\"Read Current\" pressed" ("L10n_Action 1 Pressed")) -> (w199:T56)
        n86 = call "FT10_Log Queue Data.vi"("Message Handling Cluster in"=w192) -> ("Message Handling Cluster out"=w191:T48)  [unwired: 10 in]
        n87 = Enqueue Element(queue=w203, element=w199, error in (no error)=w195) -> (error out=w202:errorcluster)  [unwired: 1 in, 2 out]
        n88 = Merge Errors(w202) -> (w197:errorcluster)
      }
      frame "7854 Set Config" {
        n89 = Variant To Data(type=T59 {"7854 Config Enum"=enum."Mono 1", "7854 Set Config"=FALSE}, Variant=w216) -> (data=w221:T59)  [unwired: 1 in, 1 out]
        n90 = Unbundle By Name(w221) -> ("7854 Config Enum"=w215:T25)
        n91 = Unbundle By Name(w219) -> ("PXI-7854R FPGA Reference"=w220:T50)
        n92 = call "FT10_FPGA_7854R Set Config.vi"("7854 Config Enum"=w215) -> ("Config string"=w206:string, "Conn2/DIO_8_15 In"=w213:bool[], "Conn2/DIO_0_7 In"=w214:bool[])  [unwired: 8 in]
        n93 = xnode "Read/Write Control"("FPGA VI Reference In"=w220, "Conn2/DIO_0_7 In"=w214, "Conn2/DIO_8_15 In"=w213) -> ("FPGA VI Reference Out"=w217:T50)  [unwired: 1 in, 1 out]
        n94 = Concatenate Strings("PXI-7854R Configuration Set to " ("Display Message"), w206) -> (w205:string)
        n95 = Bundle By Name(cluster=w219, "PXI-7854R FPGA Reference"=w217) -> (w218:T48)
        n96 = Bundle By Name(cluster=T56 {"Message"="", "Message Data"=variant} ("Message Cluster"), "Message"="Update Display", "Message Data"=w205) -> (w209:T56)
        n97 = Enqueue Element(queue=w204, element=w209, error in (no error)=w207) -> (error out=w208:errorcluster)  [unwired: 1 in, 2 out]
      }
      frame "Mono1 Cut Activate Port" {
        # "Turn power ON or OFF on MONO1 Cut Port"
        n98 = Variant To Data(type=T16 FALSE ("Mono1 Cut Activate"), Variant=w227) -> (data=w224:T16)  [unwired: 1 in, 1 out]
        n99 = Unbundle By Name(w229) -> ("Fornax Connection"=w226:refnum<k5>)
        n100 = call "FT10_Fornax Mono1 Cut Activate Port Command.vi"("Mono1 Cut Activate"=w224, "TCP Network Connection in"=w226) -> ("TCP Network Connection out"=w225:refnum<k5>)  [unwired: 9 in]
        n101 = Bundle By Name(cluster=w229, "Fornax Connection"=w225) -> (w223:T48)
        n102 = Bundle By Name(cluster=T56 {"Message"="", "Message Data"=variant} ("Message Cluster"), "Message"="Update Display", "Message Data"="\"Mono1 Cut Activate Port\" pressed" ("L10n_Action 1 Pressed")) -> (w234:T56)
        n103 = Enqueue Element(queue=w232, element=w234, error in (no error)=w231) -> (error out=w230:errorcluster)  [unwired: 1 in, 2 out]
      }
      frame "Mono2 Cut Activate Port" {
        # "Turn power ON or OFF on MONO2 Cut Port"
        n104 = Variant To Data(type=T8 FALSE ("Mono2 Cut Activate"), Variant=w242) -> (data=w237:T8)  [unwired: 1 in, 1 out]
        n105 = Unbundle By Name(w243) -> ("Fornax Connection"=w239:refnum<k5>)
        n106 = call "FT10_Fornax Mono2 Cut Activate Port Command.vi"("Mono2 Cut Activate"=w237, "TCP Network Connection in"=w239) -> ("TCP Network Connection out"=w238:refnum<k5>)  [unwired: 9 in]
        n107 = Bundle By Name(cluster=w243, "Fornax Connection"=w238) -> (w241:T48)
        n108 = Bundle By Name(cluster=T56 {"Message"="", "Message Data"=variant} ("Message Cluster"), "Message"="Update Display", "Message Data"="\"Mono2 Cut Activate Port\" pressed" ("L10n_Action 1 Pressed")) -> (w248:T56)
        n109 = Enqueue Element(queue=w246, element=w248, error in (no error)=w245) -> (error out=w244:errorcluster)  [unwired: 1 in, 2 out]
      }
      frame "Mono1 Coag Activate Port" {
        # "Turn power ON or OFF on MONO1 Coag Port"
        n110 = Variant To Data(type=T11 FALSE ("Mono1 Coag Activate"), Variant=w256) -> (data=w251:T11)  [unwired: 1 in, 1 out]
        n111 = Unbundle By Name(w257) -> ("Fornax Connection"=w253:refnum<k5>)
        n112 = call "FT10_Fornax Mono1 Coag Activate Port Command.vi"("Mono1 Coag Activate"=w251, "TCP Network Connection in"=w253) -> ("TCP Network Connection out"=w252:refnum<k5>)  [unwired: 9 in]
        n113 = Bundle By Name(cluster=w257, "Fornax Connection"=w252) -> (w255:T48)
        n114 = Bundle By Name(cluster=T56 {"Message"="", "Message Data"=variant} ("Message Cluster"), "Message"="Update Display", "Message Data"="\"Mono1 Coag Activate Port\" pressed" ("L10n_Action 1 Pressed")) -> (w262:T56)
        n115 = Enqueue Element(queue=w260, element=w262, error in (no error)=w259) -> (error out=w258:errorcluster)  [unwired: 1 in, 2 out]
      }
      frame "Mono2 Coag Activate Port" {
        # "Turn power ON or OFF on MONO2 Coag Port"
        n116 = Variant To Data(type=T4 FALSE ("Mono2 Coag Activate"), Variant=w268) -> (data=w265:T4)  [unwired: 1 in, 1 out]
        n117 = Unbundle By Name(w271) -> ("Fornax Connection"=w267:refnum<k5>)
        n118 = call "FT10_Fornax Mono2 Coag Activate Port Command.vi"("Mono2 Coag Activate"=w265, "TCP Network Connection in"=w267) -> ("TCP Network Connection out"=w266:refnum<k5>)  [unwired: 9 in]
        n119 = Bundle By Name(cluster=w271, "Fornax Connection"=w266) -> (w270:T48)
        n120 = Bundle By Name(cluster=T56 {"Message"="", "Message Data"=variant} ("Message Cluster"), "Message"="Update Display", "Message Data"="\"Mono2 Coag Activate Port\" pressed" ("L10n_Action 1 Pressed")) -> (w276:T56)
        n121 = Enqueue Element(queue=w274, element=w276, error in (no error)=w273) -> (error out=w272:errorcluster)  [unwired: 1 in, 2 out]
      }
      frame "Ligasure Activate Port" {
        # "Turn power ON or OFF on Ligasure Port"
        n122 = Variant To Data(type=T21 FALSE ("Ligasure Activate"), Variant=w282) -> (data=w279:T21)  [unwired: 1 in, 1 out]
        n123 = Unbundle By Name(w285) -> ("Fornax Connection"=w281:refnum<k5>)
        n124 = call "FT10_Fornax Ligasure Activate Port Command.vi"("Ligasure Activate"=w279, "TCP Network Connection in"=w281) -> ("TCP Network Connection out"=w280:refnum<k5>)  [unwired: 9 in]
        n125 = Bundle By Name(cluster=w285, "Fornax Connection"=w280) -> (w284:T48)
        n126 = Bundle By Name(cluster=T56 {"Message"="", "Message Data"=variant} ("Message Cluster"), "Message"="Update Display", "Message Data"="\"Ligasure Activate Port\" pressed" ("L10n_Action 1 Pressed")) -> (w290:T56)
        n127 = Enqueue Element(queue=w288, element=w290, error in (no error)=w287) -> (error out=w286:errorcluster)  [unwired: 1 in, 2 out]
      }
      frame "Bipolar Activate Port" {
        # "Turn power ON or OFF on Bipolar Port"
        n128 = Variant To Data(type=T20 FALSE ("Bipolar Activate"), Variant=w296) -> (data=w293:T20)  [unwired: 1 in, 1 out]
        n129 = Unbundle By Name(w299) -> ("Fornax Connection"=w295:refnum<k5>)
        n130 = call "FT10_Fornax Bipolar Activate Port Command.vi"("Bipolar Activate"=w293, "TCP Network Connection in"=w295) -> ("TCP Network Connection out"=w294:refnum<k5>)  [unwired: 9 in]
        n131 = Bundle By Name(cluster=w299, "Fornax Connection"=w294) -> (w298:T48)
        n132 = Bundle By Name(cluster=T56 {"Message"="", "Message Data"=variant} ("Message Cluster"), "Message"="Update Display", "Message Data"="\"Bipolar Activate Port\" pressed" ("L10n_Action 1 Pressed")) -> (w304:T56)
        n133 = Enqueue Element(queue=w302, element=w304, error in (no error)=w301) -> (error out=w300:errorcluster)  [unwired: 1 in, 2 out]
      }
      frame "Mono1 Cut Decrease Power" {
        # "Decrease Mono1 Cut Power"
        # "Turn power level down on MONO1 Cut Port"
        n134 = Unbundle By Name(w318) -> ("Fornax Connection"=w309:refnum<k5>)
        n135 = call "FT10_Fornax Energy Parameter Command.vi"("Energy Channel ID"=Control_Fornax_Energy_Channel_ID."EC_MONO_1  ", "Generator"=T65 "CAMM_EXT_1234321_AJ1428000", "Instrument Type"=Control_Fornax_Instrument_Type."INSTRUMENT_TYPE_MONOPOLAR", "Parameter Type"=Control_Fornax_Parameter_Type."CUT_MODALITY_POWER_PARAMETER", "Parameter Value"=T61 2, "Energy Mode"=Control_Fornax_Energy_Mode."CUT_MODE") -> ("JSON Command"=w307:string)  [unwired: 9 in]
        n136 = TCP Write(connection ID=w309, data in=w307, 9:100 ("timeout ms (25000)")) -> (connection ID out=w308:refnum<k5>)  [unwired: 1 in, 2 out]
        n137 = Bundle By Name(cluster=w318, "Fornax Connection"=w308) -> (w317:T48)
        n138 = Bundle By Name(cluster=T56 {"Message"="", "Message Data"=variant} ("Message Cluster"), "Message"="Update Display", "Message Data"="\"Mono1 Cut Decrease Power\" pressed" ("L10n_Action 1 Pressed")) -> (w323:T56)
        n139 = Enqueue Element(queue=w321, element=w323, error in (no error)=w320) -> (error out=w319:errorcluster)  [unwired: 1 in, 2 out]
      }
      frame "Mono2 Cut Decrease Power" {
        # "Decrease Mono2 Cut Power"
        # "Turn power level down on MONO2 Cut Port"
        n140 = Unbundle By Name(w337) -> ("Fornax Connection"=w334:refnum<k5>)
        n141 = call "FT10_Fornax Energy Parameter Command.vi"("Energy Channel ID"=Control_Fornax_Energy_Channel_ID."EC_MONO_2  ", "Generator"=T65 "CAMM_EXT_1234321_AJ1428000", "Instrument Type"=Control_Fornax_Instrument_Type."INSTRUMENT_TYPE_MONOPOLAR", "Parameter Type"=Control_Fornax_Parameter_Type."CUT_MODALITY_POWER_PARAMETER", "Parameter Value"=T61 2, "Energy Mode"=Control_Fornax_Energy_Mode."CUT_MODE") -> ("JSON Command"=w326:string)  [unwired: 9 in]
        n142 = TCP Write(connection ID=w334, data in=w326, 9:100 ("timeout ms (25000)")) -> (connection ID out=w333:refnum<k5>)  [unwired: 1 in, 2 out]
        n143 = Bundle By Name(cluster=w337, "Fornax Connection"=w333) -> (w336:T48)
        n144 = Bundle By Name(cluster=T56 {"Message"="", "Message Data"=variant} ("Message Cluster"), "Message"="Update Display", "Message Data"="\"Mono2 Cut Decrease Power\" pressed" ("L10n_Action 1 Pressed")) -> (w342:T56)
        n145 = Enqueue Element(queue=w340, element=w342, error in (no error)=w339) -> (error out=w338:errorcluster)  [unwired: 1 in, 2 out]
      }
      frame "Mono1 Coag Decrease Power" {
        # "Decrease Mono1 Coag Power"
        # "Turn power level down on MONO1 Coag Port"
        n146 = Unbundle By Name(w356) -> ("Fornax Connection"=w353:refnum<k5>)
        n147 = call "FT10_Fornax Energy Parameter Command.vi"("Energy Channel ID"=Control_Fornax_Energy_Channel_ID."EC_MONO_1  ", "Generator"=T65 "CAMM_EXT_1234321_AJ1428000", "Instrument Type"=Control_Fornax_Instrument_Type."INSTRUMENT_TYPE_MONOPOLAR", "Parameter Type"=Control_Fornax_Parameter_Type."COAG_MODALITY_POWER_PARAMETER", "Parameter Value"=T61 2, "Energy Mode"=Control_Fornax_Energy_Mode."FULGERATE_MODE") -> ("JSON Command"=w345:string)  [unwired: 9 in]
        n148 = TCP Write(connection ID=w353, data in=w345, 9:100 ("timeout ms (25000)")) -> (connection ID out=w352:refnum<k5>)  [unwired: 1 in, 2 out]
        n149 = Bundle By Name(cluster=w356, "Fornax Connection"=w352) -> (w355:T48)
        n150 = Bundle By Name(cluster=T56 {"Message"="", "Message Data"=variant} ("Message Cluster"), "Message"="Update Display", "Message Data"="\"Mono1 Coag Decrease Power\" pressed" ("L10n_Action 1 Pressed")) -> (w361:T56)
        n151 = Enqueue Element(queue=w359, element=w361, error in (no error)=w358) -> (error out=w357:errorcluster)  [unwired: 1 in, 2 out]
      }
      frame "Mono2 Coag Decrease Power" {
        # "Decrease Mono2 Coag Power"
        # "Turn power level down on MONO2 Coag Port"
        n152 = Unbundle By Name(w375) -> ("Fornax Connection"=w372:refnum<k5>)
        n153 = call "FT10_Fornax Energy Parameter Command.vi"("Energy Channel ID"=Control_Fornax_Energy_Channel_ID."EC_MONO_2  ", "Generator"=T65 "CAMM_EXT_1234321_AJ1428000", "Instrument Type"=Control_Fornax_Instrument_Type."INSTRUMENT_TYPE_MONOPOLAR", "Parameter Type"=Control_Fornax_Parameter_Type."COAG_MODALITY_POWER_PARAMETER", "Parameter Value"=T61 2, "Energy Mode"=Control_Fornax_Energy_Mode."FULGERATE_MODE") -> ("JSON Command"=w364:string)  [unwired: 9 in]
        n154 = TCP Write(connection ID=w372, data in=w364, 9:100 ("timeout ms (25000)")) -> (connection ID out=w371:refnum<k5>)  [unwired: 1 in, 2 out]
        n155 = Bundle By Name(cluster=w375, "Fornax Connection"=w371) -> (w374:T48)
        n156 = Bundle By Name(cluster=T56 {"Message"="", "Message Data"=variant} ("Message Cluster"), "Message"="Update Display", "Message Data"="\"Mono2 Coag Decrease Power\" pressed" ("L10n_Action 1 Pressed")) -> (w380:T56)
        n157 = Enqueue Element(queue=w378, element=w380, error in (no error)=w377) -> (error out=w376:errorcluster)  [unwired: 1 in, 2 out]
      }
      frame "Bipolar Decrease Power" {
        # "Decrease Bipolar Power"
        # "Turn power level down on Bipolar Port"
        n158 = Unbundle By Name(w394) -> ("Fornax Connection"=w391:refnum<k5>)
        n159 = call "FT10_Fornax Energy Parameter Command.vi"("Energy Channel ID"=Control_Fornax_Energy_Channel_ID."EC_BIPOLAR  ", "Generator"=T65 "CAMM_EXT_1234321_AJ1428000", "Instrument Type"=Control_Fornax_Instrument_Type."INSTRUMENT_TYPE_BIPOLAR", "Parameter Type"=Control_Fornax_Parameter_Type."POWER_PARAMETER", "Parameter Value"=T61 2, "Energy Mode"=Control_Fornax_Energy_Mode."BIPOLAR_MODE") -> ("JSON Command"=w383:string)  [unwired: 9 in]
        n160 = TCP Write(connection ID=w391, data in=w383, 9:100 ("timeout ms (25000)")) -> (connection ID out=w390:refnum<k5>)  [unwired: 1 in, 2 out]
        n161 = Bundle By Name(cluster=w394, "Fornax Connection"=w390) -> (w393:T48)
        n162 = Bundle By Name(cluster=T56 {"Message"="", "Message Data"=variant} ("Message Cluster"), "Message"="Update Display", "Message Data"="\"Bipolar Decrease Power\" pressed" ("L10n_Action 1 Pressed")) -> (w399:T56)
        n163 = Enqueue Element(queue=w397, element=w399, error in (no error)=w396) -> (error out=w395:errorcluster)  [unwired: 1 in, 2 out]
      }
      frame "Mono1 Cut Increase Power" {
        # "Increase Mono1 Cut Power"
        # "Turn power level up on MONO1 Cut Port"
        n164 = Unbundle By Name(w413) -> ("Fornax Connection"=w410:refnum<k5>)
        n165 = call "FT10_Fornax Energy Parameter Command.vi"("Energy Channel ID"=Control_Fornax_Energy_Channel_ID."EC_MONO_1  ", "Generator"=T65 "CAMM_EXT_1234321_AJ1428000", "Instrument Type"=Control_Fornax_Instrument_Type."INSTRUMENT_TYPE_MONOPOLAR", "Parameter Type"=Control_Fornax_Parameter_Type."CUT_MODALITY_POWER_PARAMETER", "Parameter Value"=T61 1, "Energy Mode"=Control_Fornax_Energy_Mode."CUT_MODE") -> ("JSON Command"=w402:string)  [unwired: 9 in]
        n166 = TCP Write(connection ID=w410, data in=w402, 9:100 ("timeout ms (25000)")) -> (connection ID out=w409:refnum<k5>)  [unwired: 1 in, 2 out]
        n167 = Bundle By Name(cluster=w413, "Fornax Connection"=w409) -> (w412:T48)
        n168 = Bundle By Name(cluster=T56 {"Message"="", "Message Data"=variant} ("Message Cluster"), "Message"="Update Display", "Message Data"="\"Mono1 Cut Increase Power\" pressed" ("L10n_Action 1 Pressed")) -> (w418:T56)
        n169 = Enqueue Element(queue=w416, element=w418, error in (no error)=w415) -> (error out=w414:errorcluster)  [unwired: 1 in, 2 out]
      }
      frame "Mono2 Cut Increase Power" {
        # "Increase Mono2 Cut Power"
        # "Turn power level up on MONO2 Cut Port"
        n170 = Unbundle By Name(w432) -> ("Fornax Connection"=w429:refnum<k5>)
        n171 = call "FT10_Fornax Energy Parameter Command.vi"("Energy Channel ID"=Control_Fornax_Energy_Channel_ID."EC_MONO_2  ", "Generator"=T65 "CAMM_EXT_1234321_AJ1428000", "Instrument Type"=Control_Fornax_Instrument_Type."INSTRUMENT_TYPE_MONOPOLAR", "Parameter Type"=Control_Fornax_Parameter_Type."CUT_MODALITY_POWER_PARAMETER", "Parameter Value"=T61 1, "Energy Mode"=Control_Fornax_Energy_Mode."CUT_MODE") -> ("JSON Command"=w421:string)  [unwired: 9 in]
        n172 = TCP Write(connection ID=w429, data in=w421, 9:100 ("timeout ms (25000)")) -> (connection ID out=w428:refnum<k5>)  [unwired: 1 in, 2 out]
        n173 = Bundle By Name(cluster=w432, "Fornax Connection"=w428) -> (w431:T48)
        n174 = Bundle By Name(cluster=T56 {"Message"="", "Message Data"=variant} ("Message Cluster"), "Message"="Update Display", "Message Data"="\"Mono2 Cut Increase Power\" pressed" ("L10n_Action 1 Pressed")) -> (w437:T56)
        n175 = Enqueue Element(queue=w435, element=w437, error in (no error)=w434) -> (error out=w433:errorcluster)  [unwired: 1 in, 2 out]
      }
      frame "Mono1 Coag Increase Power" {
        # "Increase Mono1 Coag Power"
        # "Turn power level up on MONO1 Coag Port"
        n176 = Unbundle By Name(w451) -> ("Fornax Connection"=w448:refnum<k5>)
        n177 = call "FT10_Fornax Energy Parameter Command.vi"("Energy Channel ID"=Control_Fornax_Energy_Channel_ID."EC_MONO_1  ", "Generator"=T65 "CAMM_EXT_1234321_AJ1428000", "Instrument Type"=Control_Fornax_Instrument_Type."INSTRUMENT_TYPE_MONOPOLAR", "Parameter Type"=Control_Fornax_Parameter_Type."COAG_MODALITY_POWER_PARAMETER", "Parameter Value"=T61 1, "Energy Mode"=Control_Fornax_Energy_Mode."FULGERATE_MODE") -> ("JSON Command"=w440:string)  [unwired: 9 in]
        n178 = TCP Write(connection ID=w448, data in=w440, 9:100 ("timeout ms (25000)")) -> (connection ID out=w447:refnum<k5>)  [unwired: 1 in, 2 out]
        n179 = Bundle By Name(cluster=w451, "Fornax Connection"=w447) -> (w450:T48)
        n180 = Bundle By Name(cluster=T56 {"Message"="", "Message Data"=variant} ("Message Cluster"), "Message"="Update Display", "Message Data"="\"Mono1 Coag Increase Power\" pressed" ("L10n_Action 1 Pressed")) -> (w456:T56)
        n181 = Enqueue Element(queue=w454, element=w456, error in (no error)=w453) -> (error out=w452:errorcluster)  [unwired: 1 in, 2 out]
      }
      frame "Mono2 Coag Increase Power" {
        # "Increase Mono2 Coag Power"
        # "Turn power level up on MONO2 Coag Port"
        n182 = Unbundle By Name(w470) -> ("Fornax Connection"=w467:refnum<k5>)
        n183 = call "FT10_Fornax Energy Parameter Command.vi"("Energy Channel ID"=Control_Fornax_Energy_Channel_ID."EC_MONO_2  ", "Generator"=T65 "CAMM_EXT_1234321_AJ1428000", "Instrument Type"=Control_Fornax_Instrument_Type."INSTRUMENT_TYPE_MONOPOLAR", "Parameter Type"=Control_Fornax_Parameter_Type."COAG_MODALITY_POWER_PARAMETER", "Parameter Value"=T61 1, "Energy Mode"=Control_Fornax_Energy_Mode."FULGERATE_MODE") -> ("JSON Command"=w459:string)  [unwired: 9 in]
        n184 = TCP Write(connection ID=w467, data in=w459, 9:100 ("timeout ms (25000)")) -> (connection ID out=w466:refnum<k5>)  [unwired: 1 in, 2 out]
        n185 = Bundle By Name(cluster=w470, "Fornax Connection"=w466) -> (w469:T48)
        n186 = Bundle By Name(cluster=T56 {"Message"="", "Message Data"=variant} ("Message Cluster"), "Message"="Update Display", "Message Data"="\"Mono2 Coag Increase Power\" pressed" ("L10n_Action 1 Pressed")) -> (w475:T56)
        n187 = Enqueue Element(queue=w473, element=w475, error in (no error)=w472) -> (error out=w471:errorcluster)  [unwired: 1 in, 2 out]
      }
      frame "Bipolar Increase Power" {
        # "Increase Bipolar Power"
        # "Turn power level up on Bipolar Port"
        n188 = Unbundle By Name(w489) -> ("Fornax Connection"=w486:refnum<k5>)
        n189 = call "FT10_Fornax Energy Parameter Command.vi"("Energy Channel ID"=Control_Fornax_Energy_Channel_ID."EC_BIPOLAR  ", "Generator"=T65 "CAMM_EXT_1234321_AJ1428000", "Instrument Type"=Control_Fornax_Instrument_Type."INSTRUMENT_TYPE_BIPOLAR", "Parameter Type"=Control_Fornax_Parameter_Type."POWER_PARAMETER", "Parameter Value"=T61 1, "Energy Mode"=Control_Fornax_Energy_Mode."BIPOLAR_MODE") -> ("JSON Command"=w478:string)  [unwired: 9 in]
        n190 = TCP Write(connection ID=w486, data in=w478, 9:100 ("timeout ms (25000)")) -> (connection ID out=w485:refnum<k5>)  [unwired: 1 in, 2 out]
        n191 = Bundle By Name(cluster=w489, "Fornax Connection"=w485) -> (w488:T48)
        n192 = Bundle By Name(cluster=T56 {"Message"="", "Message Data"=variant} ("Message Cluster"), "Message"="Update Display", "Message Data"="\"Bipolar Increase Power\" pressed" ("L10n_Action 1 Pressed")) -> (w494:T56)
        n193 = Enqueue Element(queue=w492, element=w494, error in (no error)=w491) -> (error out=w490:errorcluster)  [unwired: 1 in, 2 out]
      }
      frame "Mono1 Cut Mode" {
        # "Change mode on MONO1 Cut Port"
        n194 = Variant To Data(type=Control_Fornax_Mono1_Cut_Enum."Pure" ("Mono1 Cut Enum"), Variant=w499) -> (data=w498:T15)  [unwired: 1 in, 1 out]
        n195 = Unbundle By Name(w505) -> ("Fornax Connection"=w502:refnum<k5>)
        n196 = call "FT10_Fornax Mono1 Cut Mode Command.vi"("Mono1 Cut Enum"=w498) -> ("JSON Command"=w497:string)  [unwired: 10 in]
        n197 = TCP Write(connection ID=w502, data in=w497, 9:100 ("timeout ms (25000)")) -> (connection ID out=w501:refnum<k5>)  [unwired: 1 in, 2 out]
        n198 = Bundle By Name(cluster=w505, "Fornax Connection"=w501) -> (w504:T48)
        n199 = Bundle By Name(cluster=T56 {"Message"="", "Message Data"=variant} ("Message Cluster"), "Message"="Update Display", "Message Data"="\"Mono1 Cut Mode\" pressed" ("L10n_Action 1 Pressed")) -> (w510:T56)
        n200 = Enqueue Element(queue=w508, element=w510, error in (no error)=w507) -> (error out=w506:errorcluster)  [unwired: 1 in, 2 out]
      }
      frame "Mono2 Cut Mode" {
        # "Change mode on MONO2 Cut Port"
        n201 = Variant To Data(type=Control_Fornax_Mono2_Cut_Enum."Pure" ("Mono2 Cut Enum"), Variant=w515) -> (data=w514:T5)  [unwired: 1 in, 1 out]
        n202 = Unbundle By Name(w521) -> ("Fornax Connection"=w518:refnum<k5>)
        n203 = call "FT10_Fornax Mono2 Cut Mode Command.vi"("Mono2 Cut Enum"=w514) -> ("JSON Command"=w513:string)  [unwired: 10 in]
        n204 = TCP Write(connection ID=w518, data in=w513, 9:100 ("timeout ms (25000)")) -> (connection ID out=w517:refnum<k5>)  [unwired: 1 in, 2 out]
        n205 = Bundle By Name(cluster=w521, "Fornax Connection"=w517) -> (w520:T48)
        n206 = Bundle By Name(cluster=T56 {"Message"="", "Message Data"=variant} ("Message Cluster"), "Message"="Update Display", "Message Data"="\"Mono2 Cut Mode\" pressed" ("L10n_Action 1 Pressed")) -> (w526:T56)
        n207 = Enqueue Element(queue=w524, element=w526, error in (no error)=w523) -> (error out=w522:errorcluster)  [unwired: 1 in, 2 out]
      }
      frame "Mono1 Coag Mode" {
        # "Change mode on MONO1 Coag Port"
        n208 = Variant To Data(type=Control_Fornax_Mono1_Coag_Enum."Fulgerate" ("Mono1 Coag Enum"), Variant=w530) -> (data=w529:T12)  [unwired: 1 in, 1 out]
        n209 = Unbundle By Name(w537) -> ("Fornax Connection"=w534:refnum<k5>)
        n210 = call "FT10_Fornax Mono1 Coag Mode Command.vi"("Mono1 Coag Enum"=w529) -> ("JSON Command"=w531:string)  [unwired: 10 in]
        n211 = TCP Write(connection ID=w534, data in=w531, 9:100 ("timeout ms (25000)")) -> (connection ID out=w533:refnum<k5>)  [unwired: 1 in, 2 out]
        n212 = Bundle By Name(cluster=w537, "Fornax Connection"=w533) -> (w536:T48)
        n213 = Bundle By Name(cluster=T56 {"Message"="", "Message Data"=variant} ("Message Cluster"), "Message"="Update Display", "Message Data"="\"Mono1 Coag Mode\" pressed" ("L10n_Action 1 Pressed")) -> (w542:T56)
        n214 = Enqueue Element(queue=w540, element=w542, error in (no error)=w539) -> (error out=w538:errorcluster)  [unwired: 1 in, 2 out]
      }
      frame "Mono2 Coag Mode" {
        # "Change mode on MONO2 Coag Port"
        n215 = Variant To Data(type=Control_Fornax_Mono2_Coag_Enum."Fulgerate" ("Mono2 Coag Enum"), Variant=w547) -> (data=w546:T3)  [unwired: 1 in, 1 out]
        n216 = Unbundle By Name(w553) -> ("Fornax Connection"=w550:refnum<k5>)
        n217 = call "FT10_Fornax Mono2 Coag Mode Command.vi"("Mono2 Coag Enum"=w546) -> ("JSON Command"=w545:string)  [unwired: 10 in]
        n218 = TCP Write(connection ID=w550, data in=w545, 9:100 ("timeout ms (25000)")) -> (connection ID out=w549:refnum<k5>)  [unwired: 1 in, 2 out]
        n219 = Bundle By Name(cluster=w553, "Fornax Connection"=w549) -> (w552:T48)
        n220 = Bundle By Name(cluster=T56 {"Message"="", "Message Data"=variant} ("Message Cluster"), "Message"="Update Display", "Message Data"="\"Mono2 Coag Mode\" pressed" ("L10n_Action 1 Pressed")) -> (w558:T56)
        n221 = Enqueue Element(queue=w556, element=w558, error in (no error)=w555) -> (error out=w554:errorcluster)  [unwired: 1 in, 2 out]
      }
      frame "Bipolar Mode" {
        # "Change mode on Bipolar Port"
        n222 = Variant To Data(type=Control_Fornax_Bipolar_Enum."Standard" ("Bipolar Enum"), Variant=w563) -> (data=w562:T17)  [unwired: 1 in, 1 out]
        n223 = Unbundle By Name(w569) -> ("Fornax Connection"=w566:refnum<k5>)
        n224 = call "FT10_Fornax Bipolar Mode Command.vi"("Bipolar Enum"=w562) -> ("JSON Command"=w561:string)  [unwired: 10 in]
        n225 = TCP Write(connection ID=w566, data in=w561, 9:100 ("timeout ms (25000)")) -> (connection ID out=w565:refnum<k5>)  [unwired: 1 in, 2 out]
        n226 = Bundle By Name(cluster=w569, "Fornax Connection"=w565) -> (w568:T48)
        n227 = Bundle By Name(cluster=T56 {"Message"="", "Message Data"=variant} ("Message Cluster"), "Message"="Update Display", "Message Data"="\"Bipolar Mode\" pressed" ("L10n_Action 1 Pressed")) -> (w574:T56)
        n228 = Enqueue Element(queue=w572, element=w574, error in (no error)=w571) -> (error out=w570:errorcluster)  [unwired: 1 in, 2 out]
      }
      frame "Log?" {
        # "Update Log Flag"
        n229 = Variant To Data(type=T55 FALSE ("Log Flag"), Variant=w581) -> (data=w578:T55)  [unwired: 1 in, 1 out]
        n230 = Bundle By Name(cluster=w580, "Log Flag"=w578) -> (w579:T48)
      }
      frame "Update Display" {
        # "Update Display - Convert the Message Data to a string to display in the Display Message indicator."
        n231 = Variant To Data(error in=w588, type="", Variant=w587) -> (data=→"Display Message":string, error out=w585:errorcluster)
      }
      frame "Exit" {
        w592 = bool[] [FALSE, FALSE, FALSE, FALSE, FALSE, FALSE, FALSE, FALSE] ("Conn2/DIO_0_7 In")
        # "Release the message queue reference."
        # "Exit - Exit the application. Since this message was sent as a priority message (i.e., it was placed at the front of the queue), any cleanup code should run here, since the loop is about to stop. Any other messages in the queue will not be handled."
        n232 = Unbundle By Name(w599) -> ("UNITHERM Connection"=w601:refnum<visa-resource-name>, "PXI-7854R FPGA Reference"=w595:T50)
        n233 = xnode "Read/Write Control"("FPGA VI Reference In"=w595, "error in"=w596, "Conn2/DIO_0_7 In"=w592, "Conn2/DIO_8_15 In"=w592) -> ("FPGA VI Reference Out"=w593:T50, "error out"=w594:errorcluster)
        n234 = Release Queue(queue=w604, error in (no error)=w596) -> (error out=w603:errorcluster)  [unwired: 1 in, 2 out]
        n235 = call "FT10_Unitherm Clear Load.vi"("error in (no error)"=w596, "VISA Refnum in"=w601) -> ("error out"=w597:errorcluster, "VISA Refnum out"=w600:refnum<visa-resource-name>)  [unwired: 8 in]
        n236 = Merge Errors(w597, w594, w603) -> (w590:errorcluster)
        n237 = Bundle By Name(cluster=w599, "UNITHERM Connection"=w600, "PXI-7854R FPGA Reference"=w593) -> (w598:T48)
        n238 = flat-sequence {
          tunnel: w590 -> [w605]
          tunnel: [w605] -> w589
          frame #0 {
            n239 = call "FT10_Stop Notifier.vi"("Selector"=Config_Stop_Notifier_Enum."Notify") -> ()  [unwired: 9 in, 2 out]
          }
        }
        n240 = local write "Display Message"("\"Stop\" button pressed" ("L10n_Stop Pressed")) -> ()
      }
      frame Default {
        # "The Default case only runs if there is a message that isn't defined in any of the other cases. Generate an error if this occurs."
        n241 = xnode "Error Ring"("parameter 0"=w610) -> ("error out"=w608:errorcluster)
        n242 = call <vilib>:"Simple Error Handler.vi"("error in (no error)"=w608) -> ()  [unwired: 4 in, 5 out]
      }
    }
  }
  n243 = while {
    tunnel: w11 -> [w626]
    tunnel: w8 -> [w625]
    tunnel: [w622] -> w6
    tunnel: [w621] -> w7
    tunnel: [w619] -> _
    tunnel: w3 -> [w618]
    stop <- w628 stop-if-true
    # "Logging Loop"
    n244 = Get Queue Status(queue=w626, error in (no error)=w625) -> (queue out=w624:refnum<queue>, error out=w623:errorcluster, # elements in queue=w627:i32)  [unwired: 1 in, 5 out]
    n245 = Not Equal To 0?(x=w627) -> (x != 0?=w620:bool)
    "Logging?" <- w620
    n246 = case shown="True" w620 {
      tunnel: w624 -> [w634 w644]
      tunnel: w623 -> [w633 w643]
      tunnel: [w634 w642] -> w622
      tunnel: [w633 w641] -> w621
      tunnel: [w632 w640] -> w619
      tunnel: w618 -> [w632 w638]
      frame False {
        # "Do Nothing"
      }
      frame True {
        # "Log Values"
        n247 = Dequeue Element(queue=w644, error in (no error)=w643) -> (queue out=w642:refnum<queue>, element=w639:T44, error out=w641:errorcluster)  [unwired: 1 in, 1 out]
        n248 = call "FT10_Log LVM Values.vi"("Log Cluster in"=w639, "Log Loop Cluster in"=w638) -> ("Waveform filename"=w635:string, "Log Cluster out"=w636:T44, "Log Loop Cluster out"=w637:T40)  [unwired: 6 in, 1 out]
        n249 = call "FT10_Log TDMS Values.vi"("Waveform filename"=w635, "Log Cluster in"=w636, "Log Loop Cluster in"=w637) -> ("Log Loop Cluster out"=w640:T40)  [unwired: 7 in, 1 out]
      }
    }
    n250 = call "FT10_Stop Notifier.vi"("Selector"=Config_Stop_Notifier_Enum."Read Notifier") -> ("error out"=w629:errorcluster, "Notifier out"=w630:refnum<notifier>)  [unwired: 9 in]
    n251 = Get Notifier Status(notifier=w630, error in (no error)=w629) -> (current notification=w628:bool)  [unwired: 4 out]
  }
  n252 = while {
    tunnel: w19 -> [w647]
    tunnel: [w645] -> w28
    stop <- w646 stop-if-true
    # "Event Handling Loop"
    n253 = event shown="[29] \"Bipolar Enum\": Value Change" {
      selector: _ -> [_ _ _ _ _ _ _ _ _ _ _ _ _ _ _ _ _ _ _ _ _ _ _ _ _ _ _ _ _ _ _ _]
      dyn-events: _ -> [_ _ _ _ _ _ _ _ _ _ _ _ _ _ _ _ _ _ _ _ _ _ _ _ _ _ _ _ _ _ _ _]
      timeout: _ -> [_ _ _ _ _ _ _ _ _ _ _ _ _ _ _ _ _ _ _ _ _ _ _ _ _ _ _ _ _ _ _ _]
      tunnel: [_ _ _ _ _ _ _ _ _ _ _ _ _ _ _ _ _ _ _ _ _ _ _ _ _ _ _ _ _ _ TRUE TRUE] -> w646
      tunnel: w647 -> [w654 w663 w671 w681 w687 w702 w720 w726 w728 w748 w757 w766 w775 w784 w793 w801 w807 w813 w819 w825 w831 w837 w843 w849 w855 w861 w867 w873 w879 w885 w890 w894]
      tunnel: [w653 w662 w670 w680 w688 w701 w719 w725 w730 w749 w758 w767 w776 w785 w794 w802 w808 w814 w820 w826 w832 w838 w844 w850 w856 w862 w868 w874 w880 w886 w893 w897] -> w645
      event Value Change {
        # "Enqueue an \"Action 1\" message."
        n254 = event-data() -> ()  [unwired: 1 in, 1 out]
        n255 = case shown="True" "Fornax Connect/Disconnect" {
          tunnel: ["Connect" ("Boolean Text.Text") "Disconnect" ("Boolean Text.Text")] -> w648
          frame False {
          }
          frame True {
          }
        }
        n256 = property on="Fornax Connect/Disconnect" class="Bool (strict)"("BoolText.Text"=w648) -> ()  [unwired: 2 in, 2 out]
        n257 = Bundle By Name(cluster=T56 {"Message"="Fornax Connect/Disconnect", "Message Data"=variant} ("element"), "Message"="Fornax Connect/Disconnect", "Message Data"="Fornax Connect/Disconnect") -> (w650:T56)
        n258 = Enqueue Element(queue=w654, element=w650) -> (error out=w653:errorcluster)  [unwired: 2 in, 2 out]
      }
      event Value Change {
        # "Enqueue an \"Action 1\" message."
        n259 = event-data() -> ()  [unwired: 1 in, 1 out]
        n260 = case shown="True" "M4X Connect/Disconnect" {
          tunnel: ["Connect" ("Boolean Text.Text") "Disconnect" ("Boolean Text.Text")] -> w657
          frame False {
          }
          frame True {
          }
        }
        n261 = property on="M4X Connect/Disconnect" class="Bool (strict)"("BoolText.Text"=w657) -> ()  [unwired: 2 in, 2 out]
        n262 = Bundle By Name(cluster=T56 {"Message"="Fornax Connect/Disconnect", "Message Data"=variant} ("element"), "Message"="M4X Connect/Disconnect", "Message Data"="M4X Connect/Disconnect") -> (w659:T56)
        n263 = Enqueue Element(queue=w663, element=w659) -> (error out=w662:errorcluster)  [unwired: 2 in, 2 out]
      }
      event Value Change {
        # "Enqueue an \"Action 1\" message."
        n264 = event-data() -> ()  [unwired: 1 in, 1 out]
        n265 = Bundle By Name(cluster=T56 {"Message"="Fornax Connect/Disconnect", "Message Data"=variant} ("element"), "Message"="Log?", "Message Data"="Log?") -> (w667:T56)
        n266 = Enqueue Element(queue=w671, element=w667) -> (error out=w670:errorcluster)  [unwired: 2 in, 2 out]
      }
      event Value Change {
        # "Enqueue an \"Action 1\" message."
        n267 = event-data() -> ()  [unwired: 1 in, 1 out]
        n268 = Bundle By Name(cluster=T57 {"Unitherm Connect/Disconnect"=FALSE, "Unitherm Refnum in"=""}, "Unitherm Connect/Disconnect"="Unitherm Connect/Disconnect", "Unitherm Refnum in"="Unitherm Refnum in") -> (w676:T57)
        n269 = case shown="True" "Unitherm Connect/Disconnect" {
          tunnel: ["Connect" ("Boolean Text.Text") "Disconnect" ("Boolean Text.Text")] -> w672
          frame False {
          }
          frame True {
          }
        }
        n270 = property on="Unitherm Connect/Disconnect" class="Bool (strict)"("BoolText.Text"=w672) -> ()  [unwired: 2 in, 2 out]
        n271 = Bundle By Name(cluster=T56 {"Message"="Fornax Connect/Disconnect", "Message Data"=variant} ("element"), "Message"="Unitherm Connect/Disconnect", "Message Data"=w676) -> (w677:T56)
        n272 = Enqueue Element(queue=w681, element=w677) -> (error out=w680:errorcluster)  [unwired: 2 in, 2 out]
      }
      event Value Change {
        n273 = event-data() -> ()  [unwired: 1 in, 1 out]
        n274 = Bundle By Name(cluster=T58 {"PXI-7854R Resource"="PXI1Slot6", "75kHz"=TRUE, "uSec Off"=6, "uSec On"=7, "7854 Connect/Disconnect"=FALSE}, "7854 Connect/Disconnect"="7854 Connect/Disconnect", "75kHz"="75kHz", "uSec Off"="uSec Off", "uSec On"="uSec On", "PXI-7854R Resource"="resource name") -> (w689:T58)
        n275 = case shown="True" "7854 Connect/Disconnect" {
          tunnel: ["Connect" ("Boolean Text.Text") "Disconnect" ("Boolean Text.Text")] -> w685
          frame False {
          }
          frame True {
          }
        }
        n276 = property on="7854 Connect/Disconnect" class="Bool (strict)"("BoolText.Text"=w685) -> ()  [unwired: 2 in, 2 out]
        n277 = Bundle By Name(cluster=T56 {"Message"="Fornax Connect/Disconnect", "Message Data"=variant} ("element"), "Message"="7854 Connect/Disconnect", "Message Data"=w689) -> (w695:T56)
        n278 = Enqueue Element(queue=w687, element=w695) -> (error out=w688:errorcluster)  [unwired: 2 in, 2 out]
      }
      event Value Change {
        # "Enqueue an \"Action 1\" message."
        n279 = event-data() -> ()  [unwired: 1 in, 1 out]
        n280 = disable-structure shown="Disabled" {
          frame Disabled {
            n281 = call "FT10_Unitherm Ask Dialog - Set Load.vi"() -> ()  [unwired: 11 in, 1 out]
          }
          frame Enabled {
          }
        }
        n282 = case shown="True" "Set Load" {
          tunnel: w702 -> [w708 w714]
          tunnel: [w704 w710] -> w701
          tunnel: "Load (Ohms)" -> [w703 _]
          frame True {
            n283 = Bundle By Name(cluster=T56 {"Message"="Fornax Connect/Disconnect", "Message Data"=variant} ("element"), "Message"="Set Load", "Message Data"=w703) -> (w705:T56)
            n284 = Enqueue Element(queue=w708, element=w705) -> (error out=w704:errorcluster)  [unwired: 2 in, 2 out]
          }
          frame False {
            n285 = Bundle By Name(cluster=T56 {"Message"="Fornax Connect/Disconnect", "Message Data"=variant} ("element"), "Message"="Update Display", "Message Data"="Unitherm Set Load Canceled" ("Message")) -> (w711:T56)
            n286 = Enqueue Element(queue=w714, element=w711) -> (error out=w710:errorcluster)  [unwired: 2 in, 2 out]
          }
        }
      }
      event Value Change {
        # "Enqueue an \"Action 1\" message."
        n287 = event-data() -> ()  [unwired: 1 in, 1 out]
        n288 = Bundle By Name(cluster=T56 {"Message"="Fornax Connect/Disconnect", "Message Data"=variant} ("element"), "Message"="Clear Load", "Message Data"="Clear Load") -> (w716:T56)
        n289 = Enqueue Element(queue=w720, element=w716) -> (error out=w719:errorcluster)  [unwired: 2 in, 2 out]
      }
      event Value Change {
        # "Enqueue an \"Action 1\" message."
        n290 = event-data() -> ()  [unwired: 1 in, 1 out]
        n291 = Bundle By Name(cluster=T56 {"Message"="Fornax Connect/Disconnect", "Message Data"=variant} ("element"), "Message"="Read Current", "Message Data"="Read Current") -> (w722:T56)
        n292 = Enqueue Element(queue=w726, element=w722) -> (error out=w725:errorcluster)  [unwired: 2 in, 2 out]
      }
      event Value Change {
        n293 = event-data() -> ()  [unwired: 1 in, 1 out]
        n294 = disable-structure shown="Disabled" {
          frame Disabled {
            n295 = call "FT10_FPGA_7854R Ask Dialog - Set Config.vi"() -> ()  [unwired: 11 in, 1 out]
          }
          frame Enabled {
          }
        }
        n296 = case shown="True" "7854 Set Config" {
          selector: "7854 Set Config" -> [_ w738]
          tunnel: [w731 w740] -> w730
          tunnel: "7854 Config Enum" -> [_ w739]
          tunnel: w728 -> [w732 w737]
          frame False {
            n297 = Bundle By Name(cluster=T56 {"Message"="Fornax Connect/Disconnect", "Message Data"=variant} ("element"), "Message"="Update Display", "Message Data"="PXI-7854R Set Configuration Canceled" ("Message")) -> (w736:T56)
            n298 = Enqueue Element(queue=w732, element=w736) -> (error out=w731:errorcluster)  [unwired: 2 in, 2 out]
          }
          frame True {
            n299 = Bundle By Name(cluster=T59 {"7854 Config Enum"=enum."Mono 1", "7854 Set Config"=FALSE}, "7854 Config Enum"=w739, "7854 Set Config"=w738) -> (w741:T59)
            n300 = Bundle By Name(cluster=T56 {"Message"="Fornax Connect/Disconnect", "Message Data"=variant} ("element"), "Message"="7854 Set Config", "Message Data"=w741) -> (w744:T56)
            n301 = Enqueue Element(queue=w737, element=w744) -> (error out=w740:errorcluster)  [unwired: 2 in, 2 out]
          }
        }
      }
      event Value Change {
        # "Turn power ON or OFF on MONO1 Cut Port"
        n302 = event-data() -> ()  [unwired: 1 in, 1 out]
        n303 = case shown="True" "Mono1 Cut Activate" {
          tunnel: ["Deactivate" ("Message") "Activate" ("Message")] -> w746
          frame True {
          }
          frame False {
          }
        }
        n304 = property on="Mono1 Cut Activate" class="Bool (strict)"("BoolText.Text"=w746) -> ()  [unwired: 2 in, 2 out]
        n305 = Bundle By Name(cluster=T56 {"Message"="", "Message Data"=variant} ("element"), "Message Data"="Mono1 Cut Activate", "Message"="Mono1 Cut Activate Port") -> (w751:T56)
        n306 = Enqueue Element(queue=w748, element=w751) -> (error out=w749:errorcluster)  [unwired: 2 in, 2 out]
      }
      event Value Change {
        # "Turn power ON or OFF on MONO2 Cut Port"
        n307 = event-data() -> ()  [unwired: 1 in, 1 out]
        n308 = case shown="True" "Mono2 Cut Activate" {
          tunnel: ["Deactivate" ("Message") "Activate" ("Message")] -> w755
          frame True {
          }
          frame False {
          }
        }
        n309 = property on="Mono2 Cut Activate" class="Bool (strict)"("BoolText.Text"=w755) -> ()  [unwired: 2 in, 2 out]
        n310 = Bundle By Name(cluster=T56 {"Message"="", "Message Data"=variant} ("element"), "Message Data"="Mono2 Cut Activate", "Message"="Mono2 Cut Activate Port") -> (w760:T56)
        n311 = Enqueue Element(queue=w757, element=w760) -> (error out=w758:errorcluster)  [unwired: 2 in, 2 out]
      }
      event Value Change {
        # "Turn power ON or OFF on MONO1 Coag Port"
        n312 = event-data() -> ()  [unwired: 1 in, 1 out]
        n313 = case shown="True" "Mono1 Coag Activate" {
          tunnel: ["Deactivate" ("Message") "Activate" ("Message")] -> w764
          frame True {
          }
          frame False {
          }
        }
        n314 = property on="Mono1 Coag Activate" class="Bool (strict)"("BoolText.Text"=w764) -> ()  [unwired: 2 in, 2 out]
        n315 = Bundle By Name(cluster=T56 {"Message"="", "Message Data"=variant} ("element"), "Message Data"="Mono1 Coag Activate", "Message"="Mono1 Coag Activate Port") -> (w769:T56)
        n316 = Enqueue Element(queue=w766, element=w769) -> (error out=w767:errorcluster)  [unwired: 2 in, 2 out]
      }
      event Value Change {
        # "Turn power ON or OFF on MONO2 Coag Port"
        n317 = event-data() -> ()  [unwired: 1 in, 1 out]
        n318 = case shown="True" "Mono2 Coag Activate" {
          tunnel: ["Deactivate" ("Message") "Activate" ("Message")] -> w773
          frame True {
          }
          frame False {
          }
        }
        n319 = property on="Mono2 Coag Activate" class="Bool (strict)"("BoolText.Text"=w773) -> ()  [unwired: 2 in, 2 out]
        n320 = Bundle By Name(cluster=T56 {"Message"="", "Message Data"=variant} ("element"), "Message Data"="Mono2 Coag Activate", "Message"="Mono2 Coag Activate Port") -> (w778:T56)
        n321 = Enqueue Element(queue=w775, element=w778) -> (error out=w776:errorcluster)  [unwired: 2 in, 2 out]
      }
      event Value Change {
        # "Turn power ON or OFF on Ligasure Port"
        n322 = event-data() -> ()  [unwired: 1 in, 1 out]
        n323 = case shown="True" "Ligasure Activate" {
          tunnel: ["Deactivate" ("Message") "Activate" ("Message")] -> w783
          frame True {
          }
          frame False {
          }
        }
        n324 = property on="Ligasure Activate" class="Bool (strict)"("BoolText.Text"=w783) -> ()  [unwired: 2 in, 2 out]
        n325 = Bundle By Name(cluster=T56 {"Message"="", "Message Data"=variant} ("element"), "Message Data"="Ligasure Activate", "Message"="Ligasure Activate Port") -> (w787:T56)
        n326 = Enqueue Element(queue=w784, element=w787) -> (error out=w785:errorcluster)  [unwired: 2 in, 2 out]
      }
      event Value Change {
        # "Turn power ON or OFF on Bipolar Port"
        n327 = event-data() -> ()  [unwired: 1 in, 1 out]
        n328 = case shown="True" "Bipolar Activate" {
          tunnel: ["Deactivate" ("Message") "Activate" ("Message")] -> w792
          frame True {
          }
          frame False {
          }
        }
        n329 = property on="Bipolar Activate" class="Bool (strict)"("BoolText.Text"=w792) -> ()  [unwired: 2 in, 2 out]
        n330 = Bundle By Name(cluster=T56 {"Message"="", "Message Data"=variant} ("element"), "Message Data"="Bipolar Activate", "Message"="Bipolar Activate Port") -> (w796:T56)
        n331 = Enqueue Element(queue=w793, element=w796) -> (error out=w794:errorcluster)  [unwired: 2 in, 2 out]
      }
      event Value Change {
        # "Turn power level down on MONO1 Cut Port"
        n332 = event-data() -> ()  [unwired: 1 in, 1 out]
        n333 = Bundle By Name(cluster=T56 {"Message"="", "Message Data"=variant} ("element"), "Message Data"="Mono1 Cut minus", "Message"="Mono1 Cut Decrease Power") -> (w804:T56)
        n334 = Enqueue Element(queue=w801, element=w804) -> (error out=w802:errorcluster)  [unwired: 2 in, 2 out]
      }
      event Value Change {
        # "Turn power level down on MONO2 Cut Port"
        n335 = event-data() -> ()  [unwired: 1 in, 1 out]
        n336 = Bundle By Name(cluster=T56 {"Message"="", "Message Data"=variant} ("element"), "Message Data"="Mono2 Cut minus", "Message"="Mono2 Cut Decrease Power") -> (w810:T56)
        n337 = Enqueue Element(queue=w807, element=w810) -> (error out=w808:errorcluster)  [unwired: 2 in, 2 out]
      }
      event Value Change {
        # "Turn power level down on MONO1 Coag Port"
        n338 = event-data() -> ()  [unwired: 1 in, 1 out]
        n339 = Bundle By Name(cluster=T56 {"Message"="", "Message Data"=variant} ("element"), "Message Data"="Mono1 Coag minus", "Message"="Mono1 Coag Decrease Power") -> (w816:T56)
        n340 = Enqueue Element(queue=w813, element=w816) -> (error out=w814:errorcluster)  [unwired: 2 in, 2 out]
      }
      event Value Change {
        # "Turn power level down on MONO2 Coag Port"
        n341 = event-data() -> ()  [unwired: 1 in, 1 out]
        n342 = Bundle By Name(cluster=T56 {"Message"="", "Message Data"=variant} ("element"), "Message Data"="Mono2 Coag minus", "Message"="Mono2 Coag Decrease Power") -> (w822:T56)
        n343 = Enqueue Element(queue=w819, element=w822) -> (error out=w820:errorcluster)  [unwired: 2 in, 2 out]
      }
      event Value Change {
        # "Turn power level down on Bipolar Port"
        n344 = event-data() -> ()  [unwired: 1 in, 1 out]
        n345 = Bundle By Name(cluster=T56 {"Message"="", "Message Data"=variant} ("element"), "Message Data"="Bipolar minus", "Message"="Bipolar Decrease Power") -> (w828:T56)
        n346 = Enqueue Element(queue=w825, element=w828) -> (error out=w826:errorcluster)  [unwired: 2 in, 2 out]
      }
      event Value Change {
        # "Turn power level up on MONO1 Cut Port"
        n347 = event-data() -> ()  [unwired: 1 in, 1 out]
        n348 = Bundle By Name(cluster=T56 {"Message"="", "Message Data"=variant} ("element"), "Message Data"="Mono1 Cut plus", "Message"="Mono1 Cut Increase Power") -> (w834:T56)
        n349 = Enqueue Element(queue=w831, element=w834) -> (error out=w832:errorcluster)  [unwired: 2 in, 2 out]
      }
      event Value Change {
        # "Turn power level up on MONO2 Cut Port"
        n350 = event-data() -> ()  [unwired: 1 in, 1 out]
        n351 = Bundle By Name(cluster=T56 {"Message"="", "Message Data"=variant} ("element"), "Message Data"="Mono2 Cut plus", "Message"="Mono2 Cut Increase Power") -> (w840:T56)
        n352 = Enqueue Element(queue=w837, element=w840) -> (error out=w838:errorcluster)  [unwired: 2 in, 2 out]
      }
      event Value Change {
        # "Turn power level up on MONO1 Coag Port"
        n353 = event-data() -> ()  [unwired: 1 in, 1 out]
        n354 = Bundle By Name(cluster=T56 {"Message"="", "Message Data"=variant} ("element"), "Message Data"="Mono1 Coag plus", "Message"="Mono1 Coag Increase Power") -> (w846:T56)
        n355 = Enqueue Element(queue=w843, element=w846) -> (error out=w844:errorcluster)  [unwired: 2 in, 2 out]
      }
      event Value Change {
        # "Turn power level up on MONO2 Coag Port"
        n356 = event-data() -> ()  [unwired: 1 in, 1 out]
        n357 = Bundle By Name(cluster=T56 {"Message"="", "Message Data"=variant} ("element"), "Message Data"="Mono2 Coag plus", "Message"="Mono2 Coag Increase Power") -> (w852:T56)
        n358 = Enqueue Element(queue=w849, element=w852) -> (error out=w850:errorcluster)  [unwired: 2 in, 2 out]
      }
      event Value Change {
        # "Turn power level up on Bipolar Port"
        n359 = event-data() -> ()  [unwired: 1 in, 1 out]
        n360 = Bundle By Name(cluster=T56 {"Message"="", "Message Data"=variant} ("element"), "Message Data"="Bipolar plus", "Message"="Bipolar Increase Power") -> (w858:T56)
        n361 = Enqueue Element(queue=w855, element=w858) -> (error out=w856:errorcluster)  [unwired: 2 in, 2 out]
      }
      event Value Change {
        # "Change mode on MONO1 Cut Port"
        n362 = event-data() -> ()  [unwired: 1 in, 1 out]
        n363 = Bundle By Name(cluster=T56 {"Message"="", "Message Data"=variant} ("element"), "Message Data"="Mono1 Cut Enum", "Message"="Mono1 Cut Mode") -> (w864:T56)
        n364 = Enqueue Element(queue=w861, element=w864) -> (error out=w862:errorcluster)  [unwired: 2 in, 2 out]
      }
      event Value Change {
        # "Change mode on MONO2 Cut Port"
        n365 = event-data() -> ()  [unwired: 1 in, 1 out]
        n366 = Bundle By Name(cluster=T56 {"Message"="", "Message Data"=variant} ("element"), "Message Data"="Mono2 Cut Enum", "Message"="Mono2 Cut Mode") -> (w870:T56)
        n367 = Enqueue Element(queue=w867, element=w870) -> (error out=w868:errorcluster)  [unwired: 2 in, 2 out]
      }
      event Value Change {
        # "Change mode on MONO1 Coag Port"
        n368 = event-data() -> ()  [unwired: 1 in, 1 out]
        n369 = Bundle By Name(cluster=T56 {"Message"="", "Message Data"=variant} ("element"), "Message Data"="Mono1 Coag Enum", "Message"="Mono1 Coag Mode") -> (w876:T56)
        n370 = Enqueue Element(queue=w873, element=w876) -> (error out=w874:errorcluster)  [unwired: 2 in, 2 out]
      }
      event Value Change {
        # "Change mode on MONO2 Coag Port"
        n371 = event-data() -> ()  [unwired: 1 in, 1 out]
        n372 = Bundle By Name(cluster=T56 {"Message"="", "Message Data"=variant} ("element"), "Message Data"="Mono2 Coag Enum", "Message"="Mono2 Coag Mode") -> (w882:T56)
        n373 = Enqueue Element(queue=w879, element=w882) -> (error out=w880:errorcluster)  [unwired: 2 in, 2 out]
      }
      event Value Change {
        # "Change mode on Bipolar Port"
        n374 = event-data() -> ()  [unwired: 1 in, 1 out]
        n375 = Bundle By Name(cluster=T56 {"Message"="", "Message Data"=variant} ("element"), "Message Data"="Bipolar Enum", "Message"="Bipolar Mode") -> (w888:T56)
        n376 = Enqueue Element(queue=w885, element=w888) -> (error out=w886:errorcluster)  [unwired: 2 in, 2 out]
      }
      event Value Change {
        # "Stop the VI."
        # "Enqueue an \"Exit\" message. Note that the Enqueue Element At Opposite End function is used to place this priority \"Exit\" message at the front of the queue ahead of all other messages."
        n377 = event-data() -> ()  [unwired: 1 in, 1 out]
        n378 = Enqueue Element At Opposite End(queue=w890, element=T56 {"Message"="Exit", "Message Data"=variant}) -> (error out=w893:errorcluster)  [unwired: 2 in, 2 out]
      }
      event Panel Close? {
        # "Stop the VI."
        # "Enqueue an \"Exit\" message. Note that the Enqueue Element At Opposite End function is used to place this priority \"Exit\" message at the front of the queue ahead of all other messages."
        n379 = event-data() -> ()  [unwired: 1 in, 1 out]
        n380 = Enqueue Element At Opposite End(queue=w894, element=T56 {"Message"="Exit", "Message Data"=variant}) -> (error out=w897:errorcluster)  [unwired: 2 in, 2 out]
        n381 = event-data() -> ()  [unwired: 2 in, 1 out]
      }
    }
  }
  n382 = Release Queue(queue=w6, error in (no error)=w7) -> (error out=w5:errorcluster)  [unwired: 1 in, 2 out]
  n383 = Merge Errors(w28, w29, w5) -> (w16:errorcluster)
  n384 = call "FT10_Stop Notifier.vi"("Selector"=Config_Stop_Notifier_Enum."Close", "error in (no error)"=w16) -> ("error out"=w15:errorcluster)  [unwired: 8 in, 1 out]
  n385 = call <vilib>:"Simple Error Handler.vi"("error in (no error)"=w15) -> ()  [unwired: 4 in, 5 out]
